vi "运维调试_质控单元.vi"() -> ()   [LabVIEW 2016, in "质控单元.lvlib"]
uses:
  <vilib>/Utility/miscctls.llb/LVPointTypeDef.ctl
  <vilib>/Utility/config.llb/Write Key (I32).vi
  <vilib>/Utility/config.llb/NI_LVConfig.lvlib
panel:
  in  "适用类型":enum16{"固定站", "微站"}(ring) caption="模块组合"
  in  "模块组合":enum16{"氨氮总磷", "总磷总氮", "氨氮、总磷、总氮"}(ring)=enum."氨氮、总磷、总氮"
  in  "解锁？":bool
  in  "锁定按钮":bool
  out "模块版本号":string
  out "CODCr加标后理论浓度":dbl format="%.2f"
  out "CODMn加标后理论浓度":dbl format="%.2f"
  out "总氮加标后理论浓度":dbl format="%.2f"
  out "总磷加标后理论浓度":dbl format="%.2f"
  out "氨氮加标后理论浓度":dbl format="%.2f"
  out "CODCr母液浓度":dbl caption="加标母液浓度" format="%.2f"
  out "CODCr加标水杯定容体积":dbl caption="加标水杯定容体积" format="%.2f"
  out "CODCr检出限":dbl caption="检出限" format="%.2f"
  out "CODCr量程":dbl caption="量程" format="%.2f"
  out "COD母液浓度":dbl caption="加标母液浓度" format="%.2f"
  out "COD加标水杯定容体积":dbl caption="加标水杯定容体积" format="%.2f"
  out "COD检出限":dbl caption="检出限" format="%.2f"
  out "COD量程":dbl caption="量程" format="%.2f"
  out "总氮母液浓度":dbl caption="加标母液浓度" format="%.3f"
  out "总氮加标水杯定容体积":dbl caption="加标水杯定容体积" format="%.2f"
  out "总氮检出限":dbl caption="检出限" format="%.3f"
  out "总氮量程":dbl caption="量程" format="%.2f"
  out "总磷母液浓度":dbl caption="加标母液浓度" format="%.3f"
  out "总磷加标水杯定容体积":dbl caption="加标水杯定容体积" format="%.2f"
  out "总磷检出限":dbl caption="检出限" format="%.3f"
  out "总磷量程":dbl caption="量程" format="%.2f"
  out "氨氮母液浓度":dbl caption="加标母液浓度" format="%.3f"
  out "氨氮加标水杯定容体积":dbl caption="加标水杯定容体积" format="%.2f"
  out "氨氮检出限":dbl caption="检出限" format="%.3f"
  out "氨氮量程":dbl caption="量程" format="%.2f"
  in  "流程读写":bool
  in  "隐藏按钮":bool
  in  "定时启动":bool
  out "串口/TCP":string
  out "CODCr状态簇":T1
  out "CODMn状态簇":T1
  out "总氮状态簇":T1
  out "总磷状态簇":T1
  out "氨氮状态簇":T1
  out "总氮柱塞泵故障报警":bool
  out "总氮液位异常报警":bool
  out "总氮液位状态":bool
  out "总氮流程中断报警":bool
  out "总氮质控流程中":bool caption="总磷质控流程中"
  out "总氮通讯":bool
  out "总氮加标回收率":dbl caption="加标回收率" format="%.2f"
  out "总氮加标体积":dbl caption="加标体积" format="%.3f"
  out "总氮加标后水样浓度":dbl caption="加标后水样浓度" format="%.3f"
  out "总氮加标前水样浓度":dbl caption="加标前水样浓度" format="%.3f"
  out "总氮状态":u16(ring) caption="状态" items=["待机", "润洗", "进样", "进样完成", "柱塞泵加标", "等待取液", "排液"]
  out "CODCr柱塞泵故障报警":bool
  out "CODCr质控流程中":bool
  out "CODCr通讯":bool
  out "CODCr传感器状态":bool
  out "CODCr传感器故障报警":bool
  out "CODCr流程中断报警":bool
  out "CODCr加标回收率":dbl caption="加标回收率" format="%.2f"
  out "CODCr加标体积":dbl caption="加标体积" format="%.3f"
  out "CODCr加标后水样浓度":dbl caption="加标后水样浓度" format="%.2f"
  out "CODCr加标前水样浓度":dbl caption="加标前水样浓度" format="%.2f"
  out "CODCr状态":u16(ring) caption="状态" items=["待机", "润洗", "进样", "进样完成", "柱塞泵加标", "等待取液", "排液"]
  out "CODMn柱塞泵故障报警":bool
  out "CODMn质控流程中":bool
  out "CODMn通讯":bool
  out "CODMn液位异常报警":bool
  out "CODMn液位状态":bool
  out "CODMn流程中断报警":bool
  out "COD加标回收率":dbl caption="加标回收率" format="%.2f"
  out "COD加标体积":dbl caption="加标体积" format="%.3f"
  out "COD加标后水样浓度":dbl caption="加标后水样浓度" format="%.2f"
  out "COD加标前水样浓度":dbl caption="加标前水样浓度" format="%.2f"
  out "CODMn状态":u16(ring) caption="状态" items=["待机", "润洗", "进样", "进样完成", "柱塞泵加标", "等待取液", "排液"]
  out "总磷柱塞泵故障报警":bool
  out "总磷通讯":bool
  out "总磷质控流程中":bool caption="总氮质控流程中"
  out "总磷液位异常报警":bool
  out "总磷液位状态":bool
  out "总磷流程中断报警":bool
  out "总磷加标回收率":dbl caption="加标回收率" format="%.2f"
  out "总磷加标体积":dbl caption="加标体积" format="%.3f"
  out "总磷加标后水样浓度":dbl caption="加标后水样浓度" format="%.3f"
  out "总磷加标前水样浓度":dbl caption="加标前水样浓度" format="%.3f"
  out "总磷状态":u16(ring) caption="状态" items=["待机", "润洗", "进样", "进样完成", "柱塞泵加标", "等待取液", "排液"]
  out "氨氮柱塞泵故障报警":bool
  out "氨氮质控流程中":bool
  out "氨氮通讯":bool
  out "氨氮液位异常报警":bool
  out "氨氮液位状态":bool
  out "氨氮流程中断报警":bool
  out "氨氮加标回收率":dbl caption="加标回收率" format="%.2f"
  out "氨氮加标体积":dbl caption="加标体积" format="%.3f"
  out "氨氮加标后水样浓度":dbl caption="加标后水样浓度" format="%.3f"
  out "氨氮加标前水样浓度":dbl caption="加标前水样浓度" format="%.3f"
  out "氨氮状态":u16(ring) caption="状态" items=["待机", "润洗", "进样", "进样完成", "柱塞泵加标", "等待取液", "排液"]
  in  "总氮模块选择":bool caption="总氮模块"
  in  "释放串口":bool
  in  "打开串口":bool
  in  "柱塞泵调试":bool
  in  "手动调试":bool
  in  "报警清除":bool
  in  "参数设置":bool
  in  "停止测量":bool
  in  "加标回收":bool
  in  "平行样测试":bool
  in  "CODCr加标回收":enum32{"H", "L", "AUTO"}(ring)
  in  "CODCr选择":bool caption="CODCr模块"
  out "质控流程中":bool
  in  "CODMn加标回收":enum32{"H", "L", "AUTO"}(ring)
  in  "总磷加标回收":enum32{"H", "L", "AUTO"}(ring)=enum."AUTO"
  in  "总氮加标回收":enum32{"H", "L", "AUTO"}(ring)=enum."AUTO"
  in  "氨氮加标回收":enum32{"H", "L", "AUTO"}(ring)=enum."AUTO"
  in  "CODMn选择":bool caption="CODMn模块"
  in  "总磷模块选择":bool caption="总磷模块"
  in  "氨氮模块":bool
  in  "背隙补偿步数 3":i32 min=0 max=2000
  in  "背隙补偿步数 2":i32 min=0 max=2000
  in  "背隙补偿步数":i32 min=0 max=2000
  in  "返回":bool
  out "COD平行样测完标志":bool
  out "氨氮总磷平行样测完标志":bool
  # "氨氮"
  # "总磷"
  # "总氮"
  # "CODMn"
  # "CODCr"
  # "参数配置区"
  # "总磷质控参数"
  # "2000步等于1mL\n100步等于0.05mL\n20步等于0.01mL\n2步等于0.001mL\n（初始默认100步）"
  # "柱塞泵调试区"
  # "加标后理论浓度"
  # "mg/L"
  # "mg/L"
  # "mg/L"
  # "mg/L"
  # "mg/L"
  # "CODCr质控参数"
  # "mg/L"
  # "mL"
  # "mg/L"
  # "mg/L"
  # "CODMn质控参数"
  # "mg/L"
  # "mL"
  # "mg/L"
  # "mg/L"
  # "总氮质控参数"
  # "mg/L"
  # "mg/L"
  # "mL"
  # "mg/L"
  # "mg/L"
  # "mL"
  # "mg/L"
  # "mg/L"
  # "氨氮质控参数"
  # "mg/L"
  # "mL"
  # "mg/L"
  # "mg/L"
  # "%"
  # "mL"
  # "mg/L"
  # "mg/L"
  # "%"
  # "mL"
  # "mg/L"
  # "mg/L"
  # "%"
  # "mL"
  # "mg/L"
  # "mg/L"
  # "%"
  # "mL"
  # "mg/L"
  # "mg/L"
  # "%"
  # "mL"
  # "mg/L"
  # "mg/L"
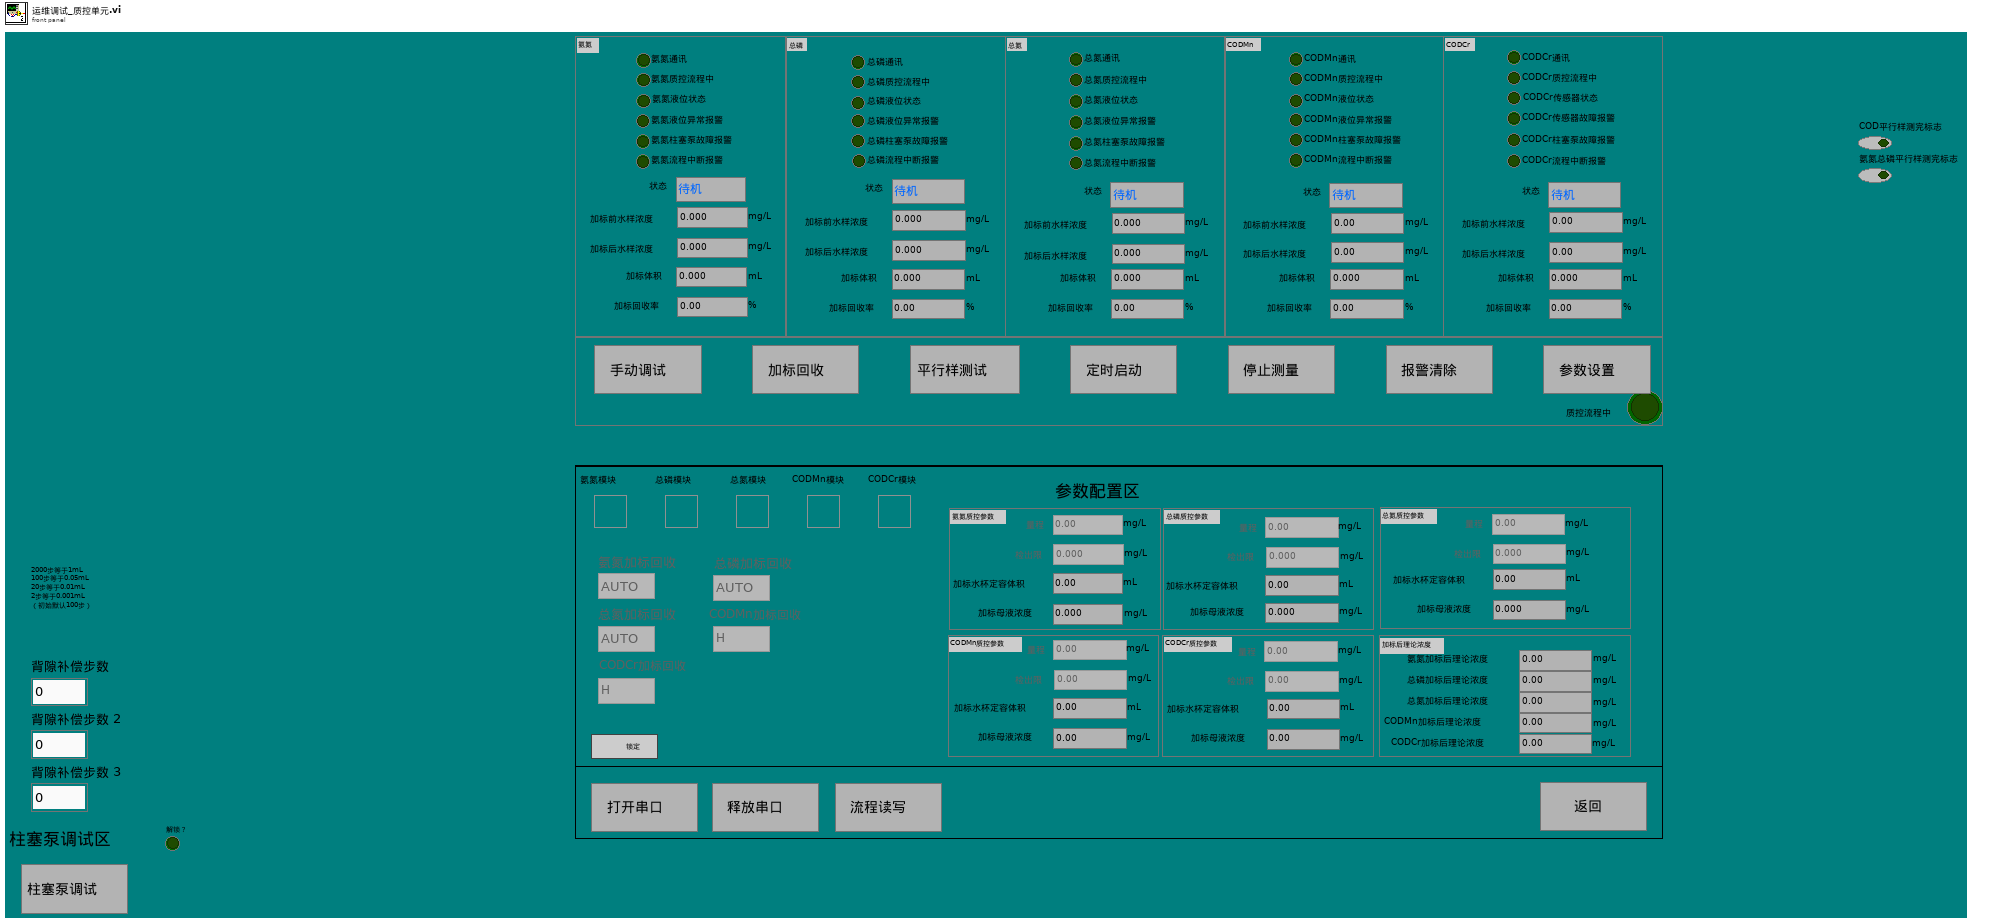
[diagram p1: front panel]
types:
  T1 = cluster{"步骤剩余时间":u16, "当前具体步骤":enum16{"加标", "进样", "排液", "搅拌", "定量"}, " 当前流程":enum16{"", "水样流程", "加标流程", "排液流程"}, "当前小步骤数":i8}
  T2 = typedef "LVPointTypeDef.ctl" = cluster{"Horizontal":i16, "Vertical":i16}
  T3 = cluster{"Major":u16, "Minor":u16, "Fix":u16, "Build":u16}
  T4 = cluster{"量程":dbl, "检出限":dbl, "加标前水样浓度":dbl, "加标后水样浓度":dbl, "加标水杯定容体积":dbl, "加标母液浓度":dbl, "加标体积":dbl, "加标回收率":dbl}
  T5 = cluster{"是否启用仪器":bool, "CODMn":cluster{"启动测量模式":cluster{"测量模式":enum16{"水样测量", "标样核查", "加标回收", "平行样", "校零", "校标"}}, "确定按钮":bool}, "启动模块":cluster{"氨氮":bool, "总磷":bool, "总氮":bool, "CODMn":bool, "CODCr":bool}, "常规启动":bool, "直接启动":bool}
  T6 = cluster{"参数启用":cluster{"CODMn":bool, "总磷":bool, "总氮":bool, "氨氮":bool, "CODcr":bool}, "采配水是否启动":bool}
  T7 = cluster{"命令":string, cluster{"starting address":u16, "holding register value":u16}}
  T8 = typedef "NI_LVConfig.lvlib/Config Data RefNum.ctl" = refnum<k1>
  T9 = cluster{"氨氮":bool, "总磷":bool, "总氮":bool, "CODMn":bool, "CODCr":bool}
  T10 = enum32{"Bad", "Idle", "Run top level", "Running"}
  T11 = cluster{"CODMn":bool, "总磷":bool, "总氮":bool, "氨氮":bool, "CODCr":bool}
  T12 = cluster{"周期设置类型":enum16{"定点启动", "间隔启动"}, "定时功能启用":bool, "定时间隔":dbl, "间隔启动次数 ":dbl, "已经启动次数 ":dbl, "24H周期设置":bool[], "模块选择":cluster{"氨氮":bool, "总磷":bool, "总氮":bool, "CODMn":bool, "CODCr":bool}, "采配水启用":bool}
  T13 = cluster{"周期设置类型":enum16{"定点启动", "间隔启动"}, "定时功能启用":bool, "定时间隔":dbl, "间隔启动次数":dbl, "已经启动次数":dbl, "24H周期设置":bool[], "模块选择":cluster{"氨氮":bool, "总磷":bool, "总氮":bool, "CODMn":bool, "CODCr":bool}, "采配水启用":bool}
  T14 = cluster{"氨氮":u8, "总磷":u8, "总氮":u8, "CODMn":u8, "CODCr":u8}
  T15 = enum8{"Enabled", "Disabled", "Disabled and Grayed Out"}
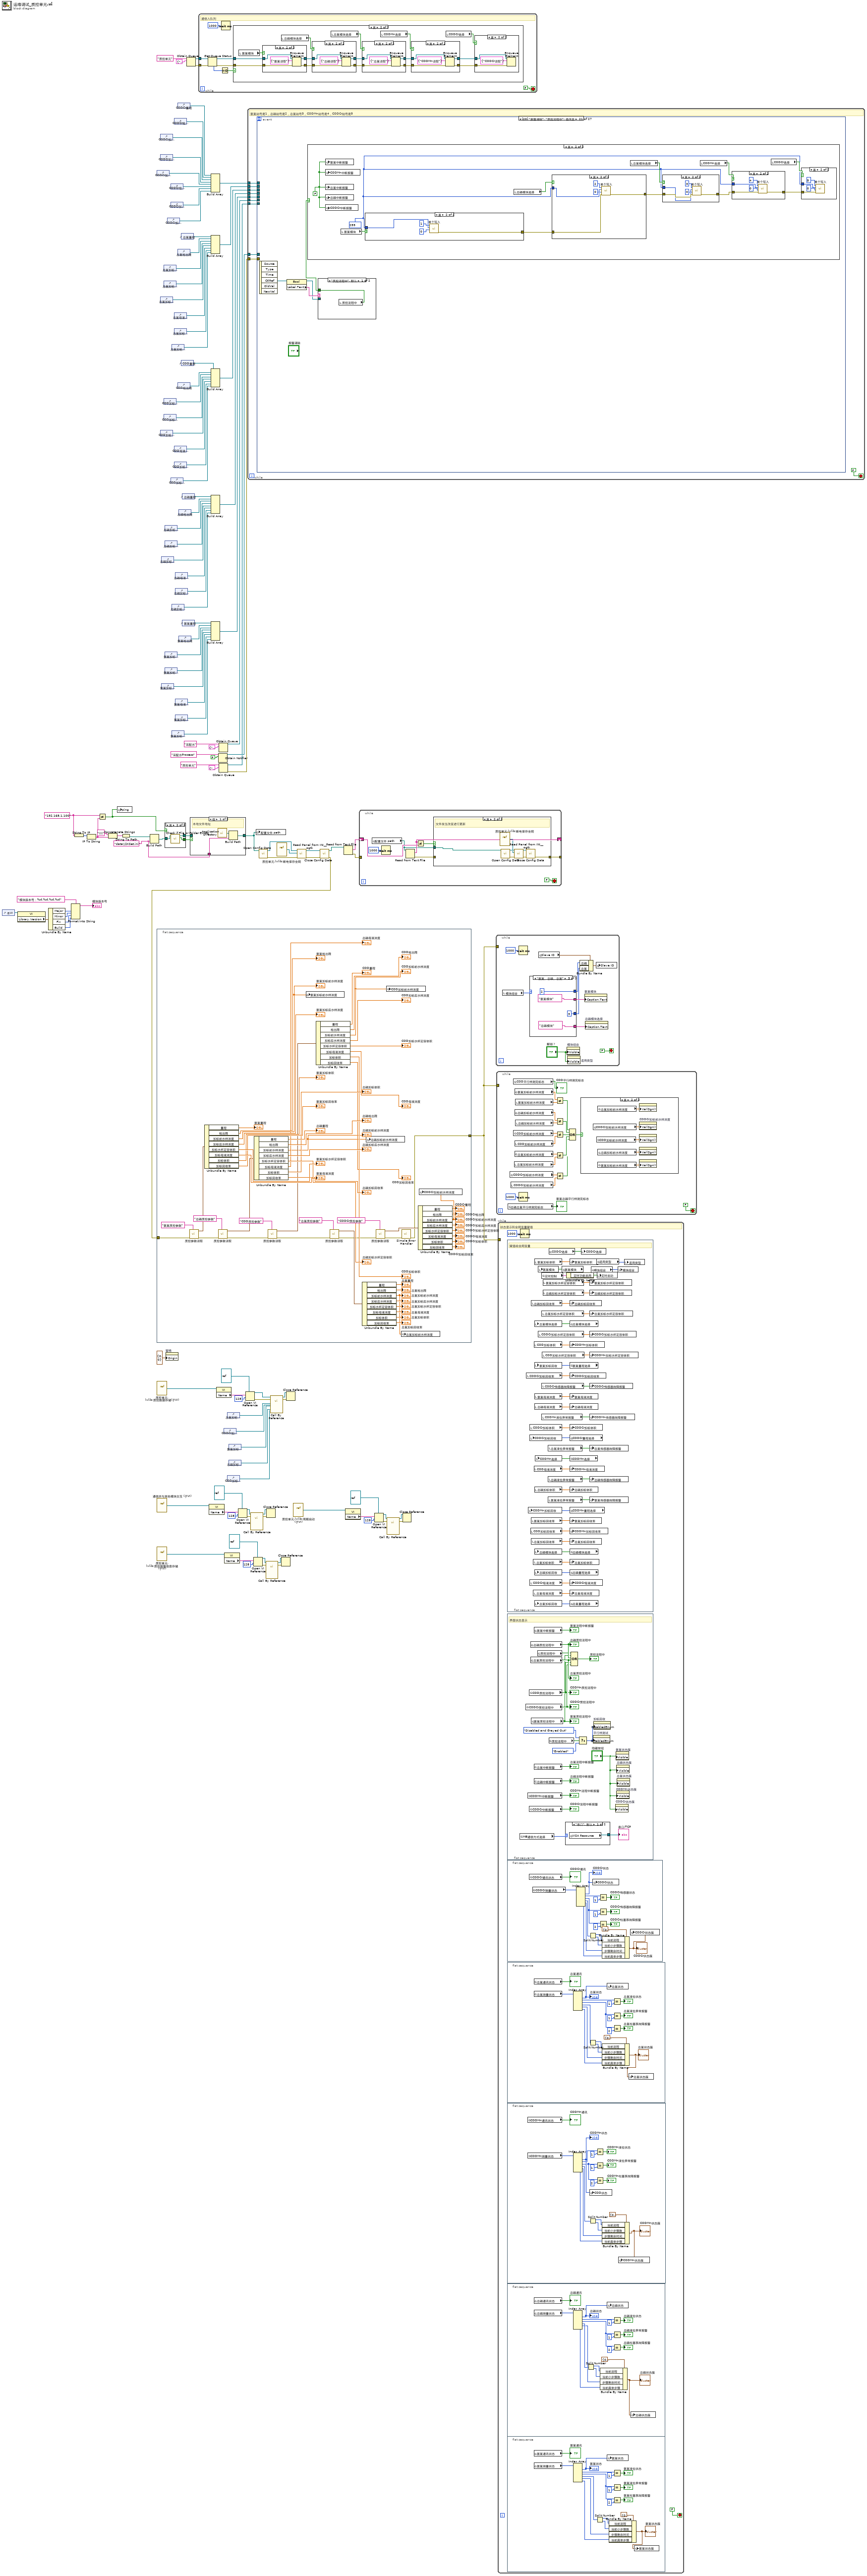
[diagram p0: block diagram]
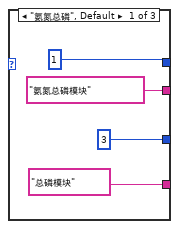
[diagram p2: hidden frame]
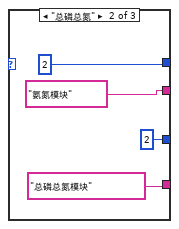
[diagram p3: hidden frame]
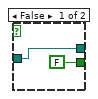
[diagram p4: hidden frame]
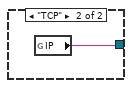
[diagram p13: hidden frame]
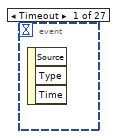
[diagram p15: hidden frame]
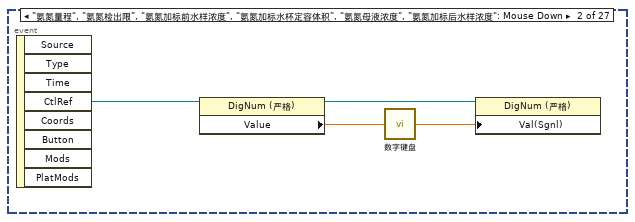
[diagram p16: hidden frame]
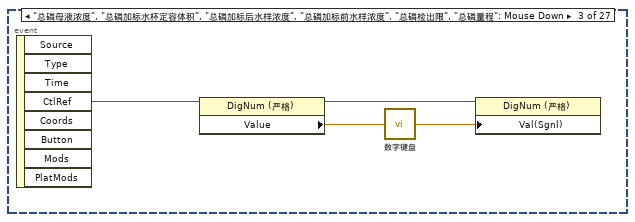
[diagram p17: hidden frame]
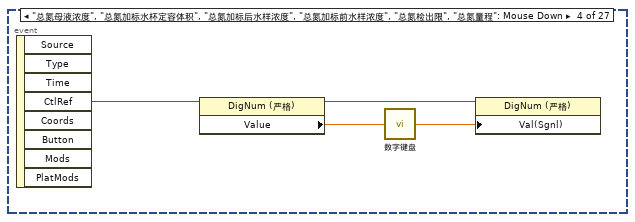
[diagram p18: hidden frame]
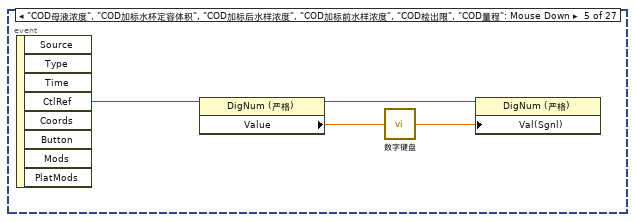
[diagram p19: hidden frame]
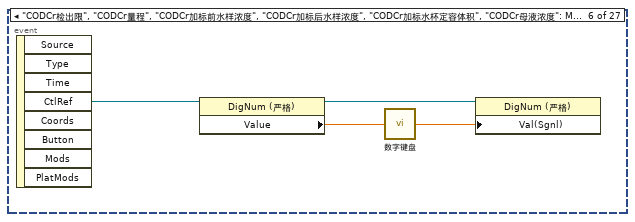
[diagram p20: hidden frame]
diagram:
  w30 = "data\\ZKSet.ini" ("名称或相对路径")
  w22 = "192.168.1.100" ("名称")
  n1 = control-ref of="本VI"() -> (w12:refnum<vi>)
  n2 = property class="VI"(reference=w12) -> ("Library.Version"=w11:T3)  [unwired: 1 in, 2 out]
  n3 = Unbundle By Name(w11) -> ("Major"=w9:u16, "Minor"=w8:u16, "Fix"=w7:u16, "Build"=w6:u16)
  n4 = Format Into String(format string="模块版本号：%d.%d.%d.%d" ("格式字符串"), w9, w8, w7, w6) -> (resulting string=→"模块版本号":string)  [unwired: 2 in, 1 out]
  n5 = String To IP(1:w22) -> (0:w29:u32)
  n6 = IP To String(2:w29) -> (0:w26:string)  [unwired: 1 in]
  n7 = Not Equal?(x=w22, y=w26) -> (x != y?=w21:bool)
  n8 = Concatenate Strings("\\\\" ("字符串"), w26) -> (w27:string)
  n9 = global write "质控内部交互全局.vi" "ping"(w21) -> ()
  n10 = String To Path(string=w27) -> (path=w3:path)
  n11 = Build Path(base path=w3, name or relative path=w30) -> (appended path=w25:path)
  n12 = control-ref of="CODCr加标水杯定容体积"() -> (w80:refnum<vi>)
  n13 = flat-sequence {
    tunnel: [w129] -> w1
    tunnel: w2 -> [w128]
    frame #0 {
      n14 = call "质控参数读取.vi"("section"="氨氮质控参数", "error in (no error)"=w128) -> ("error out"=w166:errorcluster, "参数"=w183:T4)  [unwired: 8 in]
      n15 = Unbundle By Name(w183) -> ("量程"=→"氨氮量程":dbl, "检出限"=→"氨氮检出限":dbl, "加标前水样浓度"=w134:dbl, "加标后水样浓度"=→"氨氮加标后水样浓度":dbl, "加标水杯定容体积"=→"氨氮加标水杯定容体积":dbl, "加标母液浓度"=→"氨氮母液浓度":dbl, "加标体积"=→"氨氮加标体积":dbl, "加标回收率"=→"氨氮加标回收率":dbl)
      "氨氮加标前水样浓度" <- w134
      n16 = call "质控参数读取.vi"("section"="总磷质控参数", "error in (no error)"=w166) -> ("error out"=w163:errorcluster, "参数"=w174:T4)  [unwired: 8 in]
      n17 = Unbundle By Name(w174) -> ("量程"=→"总磷量程":dbl, "检出限"=→"总磷检出限":dbl, "加标前水样浓度"=w133:dbl, "加标后水样浓度"=→"总磷加标后水样浓度":dbl, "加标水杯定容体积"=→"总磷加标水杯定容体积":dbl, "加标母液浓度"=→"总磷母液浓度":dbl, "加标体积"=→"总磷加标体积":dbl, "加标回收率"=→"总磷加标回收率":dbl)
      "总磷加标前水样浓度" <- w133
      n18 = call "质控参数读取.vi"("section"="COD质控参数", "error in (no error)"=w163) -> ("error out"=w154:errorcluster, "参数"=w165:T4)  [unwired: 8 in]
      n19 = global write "水样浓度全局.vi" "氨氮加标前水样浓度"(w134) -> ()
      n20 = Unbundle By Name(w165) -> ("量程"=→"COD量程":dbl, "检出限"=→"COD检出限":dbl, "加标前水样浓度"=w132:dbl, "加标后水样浓度"=→"COD加标后水样浓度":dbl, "加标水杯定容体积"=→"COD加标水杯定容体积":dbl, "加标母液浓度"=→"COD母液浓度":dbl, "加标体积"=→"COD加标体积":dbl, "加标回收率"=→"COD加标回收率":dbl)
      "COD加标前水样浓度" <- w132
      n21 = call "质控参数读取.vi"("section"="总氮质控参数", "error in (no error)"=w154) -> ("error out"=w143:errorcluster, "参数"=w153:T4)  [unwired: 8 in]
      n22 = Unbundle By Name(w153) -> ("量程"=→"总氮量程":dbl, "检出限"=→"总氮检出限":dbl, "加标前水样浓度"=w131:dbl, "加标后水样浓度"=→"总氮加标后水样浓度":dbl, "加标水杯定容体积"=→"总氮加标水杯定容体积":dbl, "加标母液浓度"=→"总氮母液浓度":dbl, "加标体积"=→"总氮加标体积":dbl, "加标回收率"=→"总氮加标回收率":dbl)
      "总氮加标前水样浓度" <- w131
      n23 = global write "水样浓度全局.vi" "总磷加标前水样浓度"(w133) -> ()
      n24 = call "质控参数读取.vi"("section"="CODCr质控参数", "error in (no error)"=w143) -> ("error out"=w135:errorcluster, "参数"=w144:T4)  [unwired: 8 in]
      n25 = global write "水样浓度全局.vi" "COD加标前水样浓度"(w132) -> ()
      n26 = global write "水样浓度全局.vi" "总氮加标前水样浓度"(w131) -> ()
      n27 = call <vilib>:"Simple Error Handler.vi"("error in (no error)"=w135) -> ("error out"=w129:errorcluster)  [unwired: 4 in, 4 out]
      n28 = Unbundle By Name(w144) -> ("量程"=→"CODCr量程":dbl, "检出限"=→"CODCr检出限":dbl, "加标前水样浓度"=w130:dbl, "加标后水样浓度"=→"CODCr加标后水样浓度":dbl, "加标水杯定容体积"=→"CODCr加标水杯定容体积":dbl, "加标母液浓度"=→"CODCr母液浓度":dbl, "加标体积"=→"CODCr加标体积":dbl, "加标回收率"=→"CODCr加标回收率":dbl)
      "CODCr加标前水样浓度" <- w130
      n29 = global write "水样浓度全局.vi" "CODCr加标前水样浓度"(w130) -> ()
    }
  }
  n30 = vi-ref "质控单元.lvlib:质控数据存储(子VI).vi"() -> (w55:refnum<vi>)
  n31 = vi-ref "通信并与其他模块交互 (子VI).vi"() -> (w68:refnum<vi>)
  n32 = vi-ref "质控单元.lvlib:质控报警信息存储 (子VI).vi"() -> (w63:refnum<vi>)
  n33 = control-ref of="CODCr加标前水样浓度"() -> (w82:refnum<vi>)
  n34 = control-ref of="CODCr加标后水样浓度"() -> (w81:refnum<vi>)
  n35 = control-ref of="总氮加标水杯定容体积"() -> (w89:refnum<vi>)
  n36 = control-ref of="COD加标水杯定容体积"() -> (w104:refnum<vi>)
  n37 = control-ref of="总磷加标水杯定容体积"() -> (w113:refnum<vi>)
  n38 = control-ref of="氨氮加标水杯定容体积"() -> (w123:refnum<vi>)
  n39 = control-ref of="总氮加标前水样浓度"() -> (w91:refnum<vi>)
  n40 = control-ref of="总氮加标后水样浓度"() -> (w90:refnum<vi>)
  n41 = control-ref of="COD加标前水样浓度"() -> (w106:refnum<vi>)
  n42 = control-ref of="COD加标后水样浓度"() -> (w105:refnum<vi>)
  n43 = control-ref of="总磷加标前水样浓度"() -> (w115:refnum<vi>)
  n44 = control-ref of="总磷加标后水样浓度"() -> (w114:refnum<vi>)
  n45 = control-ref of="氨氮加标前水样浓度"() -> (w124:refnum<vi>)
  n46 = control-ref of="氨氮加标后水样浓度"() -> (w120:refnum<vi>)
  n47 = case shown="真" w21 {
    tunnel: w25 -> [w185 w189]
    tunnel: [w185 w188] -> w24
    tunnel: [FALSE w187] -> w23
    frame False {
    }
    frame True {
      n48 = call <vilib>:"Check if File or Folder Exists.vi"("path"=w189) -> ("file or folder exists?"=w187:bool, "dup path"=w188:path)  [unwired: 8 in, 1 out]
    }
  }
  n49 = property on="窗格" class="Pane"("Origin"=T2 {"Horizontal"=0, "Vertical"=0} ("原点")) -> ()  [unwired: 2 in, 2 out]
  n50 = control-ref of="CODCr加标回收率"() -> (w77:refnum<vi>)
  n51 = control-ref of="CODCr母液浓度"() -> (w79:refnum<vi>)
  n52 = control-ref of="CODCr加标体积"() -> (w78:refnum<vi>)
  n53 = control-ref of="COD加标回收率"() -> (w101:refnum<vi>)
  n54 = control-ref of="总氮加标回收率"() -> (w86:refnum<vi>)
  n55 = control-ref of="总磷加标回收率"() -> (w111:refnum<vi>)
  n56 = control-ref of="氨氮加标回收率"() -> (w118:refnum<vi>)
  n57 = control-ref of="CODCr检出限"() -> (w83:refnum<vi>)
  n58 = control-ref of="总氮母液浓度"() -> (w88:refnum<vi>)
  n59 = control-ref of="总氮加标体积"() -> (w87:refnum<vi>)
  n60 = control-ref of="COD母液浓度"() -> (w103:refnum<vi>)
  n61 = control-ref of="COD加标体积"() -> (w102:refnum<vi>)
  n62 = control-ref of="总磷母液浓度"() -> (w112:refnum<vi>)
  n63 = control-ref of="总磷加标体积"() -> (w110:refnum<vi>)
  n64 = control-ref of="氨氮母液浓度"() -> (w122:refnum<vi>)
  n65 = control-ref of="氨氮加标体积"() -> (w119:refnum<vi>)
  n66 = control-ref of="CODCr量程"() -> (w84:refnum<vi>)
  n67 = control-ref of="总氮检出限"() -> (w92:refnum<vi>)
  n68 = control-ref of="COD检出限"() -> (w107:refnum<vi>)
  n69 = control-ref of="总磷检出限"() -> (w116:refnum<vi>)
  n70 = control-ref of="氨氮检出限"() -> (w125:refnum<vi>)
  n71 = control-ref of="总氮量程"() -> (w93:refnum<vi>)
  n72 = control-ref of="COD量程"() -> (w108:refnum<vi>)
  n73 = control-ref of="总磷量程"() -> (w117:refnum<vi>)
  n74 = control-ref of="氨氮量程"() -> (w126:refnum<vi>)
  n75 = Obtain Queue(name (unnamed)="质控单元" ("名称（未命名）"), element data type=cluster{"命令":string} {"命令"="启用模块"} ("元素")) -> (queue out=w40:refnum<queue>, error out=w39:errorcluster)  [unwired: 3 in, 1 out]
  n76 = case shown="假" w23 {
    tunnel: w24 -> [_ w193]
    tunnel: [w191 w193] -> w14
    tunnel: w30 -> [w190 _]
    frame False {
      # "本地文件地址"
      n77 = call <vilib>:"Application Directory.vi"() -> ("Application Directory"=w192:path)
      n78 = Build Path(base path=w192, name or relative path=w190) -> (appended path=w191:path)
    }
    frame True {
      # "网络共享地址"
    }
  }
  n79 = while {
    tunnel: w40 -> [w199]
    tunnel: w39 -> [w198]
    stop <- FALSE stop-if-true
    # "通信入队列"
    n80 = Get Queue Status(queue=w199, error in (no error)=w198) -> (queue out=w196:refnum<queue>, error out=w195:errorcluster, # elements in queue=w197:i32)  [unwired: 1 in, 5 out]
    n81 = Equal To 0?(x=w197) -> (x = 0?=w194:bool)
    n82 = Wait (ms)(milliseconds to wait=u32 1000 ("等待时间（毫秒）")) -> ()  [unwired: 1 out]
    n83 = case shown="真" w194 {
      tunnel: w196 -> [_ w216]
      tunnel: w195 -> [_ w215]
      frame False {
      }
      frame True {
        n84 = local read "氨氮模块"() -> (w214:bool)
        n85 = case shown="真" w214 {
          tunnel: w216 -> [w242 w246]
          tunnel: w215 -> [w241 w245]
          tunnel: [w242 w244] -> w212
          tunnel: [w241 w243] -> w211
          frame False {
          }
          frame True {
            n86 = Enqueue Element(queue=w246, element=cluster{"命令":string} {"命令"="氨氮读取"} ("元素"), error in (no error)=w245) -> (queue out=w244:refnum<queue>, error out=w243:errorcluster)  [unwired: 1 in, 1 out]
          }
        }
        n87 = local read "总磷模块选择"() -> (w213:bool)
        n88 = case shown="真" w213 {
          tunnel: w212 -> [w235 w239]
          tunnel: w211 -> [w234 w238]
          tunnel: [w235 w237] -> w209
          tunnel: [w234 w236] -> w208
          frame False {
          }
          frame True {
            n89 = Enqueue Element(queue=w239, element=cluster{"命令":string} {"命令"="总磷读取"} ("元素"), error in (no error)=w238) -> (queue out=w237:refnum<queue>, error out=w236:errorcluster)  [unwired: 1 in, 1 out]
          }
        }
        n90 = local read "总氮模块选择"() -> (w210:bool)
        n91 = case shown="真" w210 {
          tunnel: w209 -> [w228 w232]
          tunnel: w208 -> [w227 w231]
          tunnel: [w228 w230] -> w206
          tunnel: [w227 w229] -> w205
          frame False {
          }
          frame True {
            n92 = Enqueue Element(queue=w232, element=cluster{"命令":string} {"命令"="总氮读取"} ("元素"), error in (no error)=w231) -> (queue out=w230:refnum<queue>, error out=w229:errorcluster)  [unwired: 1 in, 1 out]
          }
        }
        n93 = local read "CODMn选择"() -> (w207:bool)
        n94 = case shown="真" w207 {
          tunnel: w206 -> [w221 w225]
          tunnel: w205 -> [w220 w224]
          tunnel: [w221 w223] -> w203
          tunnel: [w220 w222] -> w202
          frame False {
          }
          frame True {
            n95 = Enqueue Element(queue=w225, element=cluster{"命令":string} {"命令"="CODMn读取"} ("元素"), error in (no error)=w224) -> (queue out=w223:refnum<queue>, error out=w222:errorcluster)  [unwired: 1 in, 1 out]
          }
        }
        n96 = local read "CODCr选择"() -> (w204:bool)
        n97 = case shown="真" w204 {
          tunnel: w203 -> [_ w218]
          tunnel: w202 -> [_ w217]
          frame False {
          }
          frame True {
            n98 = Enqueue Element(queue=w218, element=cluster{"命令":string} {"命令"="CODCr读取"} ("元素"), error in (no error)=w217) -> ()  [unwired: 1 in, 3 out]
          }
        }
      }
    }
  }
  n99 = property class="VI"(reference=w68) -> ("Name"=w69:string)  [unwired: 1 in, 2 out]
  n100 = Build Array(w84, w83, w82, w81, w80, w79, w78, w77) -> (w76:refnum<vi>[])
  n101 = Build Array(w93, w92, w91, w90, w89, w88, w87, w86) -> (w85:refnum<vi>[])
  n102 = Build Array(w108, w107, w106, w105, w104, w103, w102, w101) -> (w100:refnum<vi>[])
  n103 = Build Array(w117, w116, w115, w114, w113, w112, w110, w111) -> (w109:refnum<vi>[])
  n104 = Build Array(w126, w125, w124, w120, w123, w122, w119, w118) -> (w121:refnum<vi>[])
  n105 = property class="VI"(reference=w55) -> ("Name"=w54:string)  [unwired: 1 in, 2 out]
  n106 = Obtain Notifier(name (unnamed)="采配水Process" ("名称（未命名）"), notification data type=FALSE) -> (notifier out=w97:refnum<notifier>)  [unwired: 2 in, 2 out]
  n107 = Obtain Queue(name (unnamed)="采配水" ("名称（未命名）"), element data type=cluster{"命令":string, "数据":variant} {"命令"="", "数据"=variant}) -> (queue out=w94:refnum<queue>)  [unwired: 3 in, 2 out]
  n108 = Obtain Queue(name (unnamed)="质控单元" ("名称（未命名）"), element data type=cluster{"命令":string} {"命令"="启用模块"} ("元素")) -> (queue out=w65:refnum<queue>, error out=w64:errorcluster)  [unwired: 3 in, 1 out]
  n109 = control-ref of="CODCr加标后水样浓度"() -> (w43:refnum<vi>)
  n110 = property class="VI"(reference=w63) -> ("Name"=w62:string)  [unwired: 1 in, 2 out]
  n111 = control-ref of="总氮加标后水样浓度"() -> (w47:refnum<vi>)
  n112 = control-ref of="COD加标后水样浓度"() -> (w44:refnum<vi>)
  n113 = control-ref of="氨氮加标后水样浓度"() -> (w46:refnum<vi>)
  n114 = control-ref of="总磷加标后水样浓度"() -> (w45:refnum<vi>)
  n115 = Open VI Reference(type specifier VI Refnum (for type only)=refnum<vi> refnum, vi path=w69, options=128 ("选项")) -> (vi reference=w71:refnum<vi>, error out=w73:errorcluster)  [unwired: 3 in]
  n116 = Open VI Reference(type specifier VI Refnum (for type only)=refnum<vi> refnum, vi path=w54, options=128 ("选项")) -> (vi reference=w52:refnum<vi>, error out=w50:errorcluster)  [unwired: 3 in]
  n117 = while {
    tunnel: w121 -> [w256]
    tunnel: w109 -> [w255]
    tunnel: w100 -> [w250]
    tunnel: w97 -> [w254]
    tunnel: w94 -> [w253]
    tunnel: w85 -> [w252]
    tunnel: w76 -> [w251]
    tunnel: w65 -> [w249]
    tunnel: w64 -> [w248]
    stop <- FALSE stop-if-true
    # "氨氮站号是1，总磷站号是2，总氮站号3，CODMn站号是4，CODCr站号是5"
    n118 = event shown="[20] \"报警清除\", \"质控流程中\": 值改变" {
      selector: _ -> [_ _ _ _ _ _ _ _ _ _ _ _ _ _ _ _ _ _ _ _ _ _ _ _ _ _ _]
      dyn-events: _ -> [_ _ _ _ _ _ _ _ _ _ _ _ _ _ _ _ _ _ _ _ _ _ _ _ _ _ _]
      timeout: _ -> [_ _ _ _ _ _ _ _ _ _ _ _ _ _ _ _ _ _ _ _ _ _ _ _ _ _ _]
      tunnel: w256 -> [_ _ _ _ _ _ _ _ _ w312 _ _ _ _ _ _ _ _ _ _ _ _ _ _ _ _ _]
      tunnel: w255 -> [_ _ _ _ _ _ _ _ _ _ w327 _ _ _ _ _ _ _ _ _ _ _ _ _ _ _ _]
      tunnel: w250 -> [_ _ _ _ _ _ _ _ _ _ _ _ w367 _ _ _ _ _ _ _ _ _ _ _ _ _ _]
      tunnel: w254 -> [_ _ _ _ _ _ _ _ _ _ _ _ _ _ _ _ _ _ _ w446 _ w527 w543 _ _ _ _]
      tunnel: w253 -> [_ _ _ _ _ _ _ _ _ _ _ _ _ _ _ _ _ _ _ _ _ _ w544 _ _ _ _]
      tunnel: w252 -> [_ _ _ _ _ _ _ _ _ _ _ w346 _ _ _ _ _ _ _ _ _ _ _ _ _ _ _]
      tunnel: w251 -> [_ _ _ _ _ _ _ _ _ _ _ _ _ w386 _ _ _ _ _ _ _ _ _ _ _ _ _]
      tunnel: w249 -> [_ _ _ _ _ _ _ _ _ _ _ _ _ _ _ _ _ w410 w430 _ _ _ _ _ _ _ _]
      tunnel: w248 -> [_ _ _ _ _ _ _ _ _ _ _ _ _ _ _ _ _ w409 w429 _ _ _ _ _ _ _ _]
      event Timeout {
        n119 = event-data() -> ()  [unwired: 1 in, 3 out]
      }
      event "氨氮量程", "氨氮检出限", "氨氮加标前水样浓度", "氨氮加标水杯定容体积", "氨氮母液浓度", "氨氮加标后水样浓度": Mouse Down {
        n120 = event-data() -> ("CtlRef"=w261:refnum<vi>)  [unwired: 1 in, 7 out]
        n121 = property class="DigNum (严格)"(reference=w261) -> (reference out=w259:refnum<vi>, "Value"=w260:dbl)  [unwired: 1 in, 1 out]
        n122 = call "数字键盘.vi"("OldNumber"=w260) -> ("NewNumber"=w258:sgl)
        n123 = property class="DigNum (严格)"(reference=w259, "Val(Sgnl)"=w258) -> ()  [unwired: 1 in, 2 out]
      }
      event "总磷母液浓度", "总磷加标水杯定容体积", "总磷加标后水样浓度", "总磷加标前水样浓度", "总磷检出限", "总磷量程": Mouse Down {
        n124 = event-data() -> ("CtlRef"=w265:refnum<vi>)  [unwired: 1 in, 7 out]
        n125 = property class="DigNum (严格)"(reference=w265) -> (reference out=w263:refnum<vi>, "Value"=w264:dbl)  [unwired: 1 in, 1 out]
        n126 = call "数字键盘.vi"("OldNumber"=w264) -> ("NewNumber"=w262:sgl)
        n127 = property class="DigNum (严格)"(reference=w263, "Val(Sgnl)"=w262) -> ()  [unwired: 1 in, 2 out]
      }
      event "总氮母液浓度", "总氮加标水杯定容体积", "总氮加标后水样浓度", "总氮加标前水样浓度", "总氮检出限", "总氮量程": Mouse Down {
        n128 = event-data() -> ("CtlRef"=w269:refnum<vi>)  [unwired: 1 in, 7 out]
        n129 = property class="DigNum (严格)"(reference=w269) -> (reference out=w267:refnum<vi>, "Value"=w268:dbl)  [unwired: 1 in, 1 out]
        n130 = call "数字键盘.vi"("OldNumber"=w268) -> ("NewNumber"=w266:sgl)
        n131 = property class="DigNum (严格)"(reference=w267, "Val(Sgnl)"=w266) -> ()  [unwired: 1 in, 2 out]
      }
      event "COD母液浓度", "COD加标水杯定容体积", "COD加标后水样浓度", "COD加标前水样浓度", "COD检出限", "COD量程": Mouse Down {
        n132 = event-data() -> ("CtlRef"=w273:refnum<vi>)  [unwired: 1 in, 7 out]
        n133 = property class="DigNum (严格)"(reference=w273) -> (reference out=w271:refnum<vi>, "Value"=w272:dbl)  [unwired: 1 in, 1 out]
        n134 = call "数字键盘.vi"("OldNumber"=w272) -> ("NewNumber"=w270:sgl)
        n135 = property class="DigNum (严格)"(reference=w271, "Val(Sgnl)"=w270) -> ()  [unwired: 1 in, 2 out]
      }
      event "CODCr检出限", "CODCr量程", "CODCr加标前水样浓度", "CODCr加标后水样浓度", "CODCr加标水杯定容体积", "CODCr母液浓度": Mouse Down {
        n136 = event-data() -> ("CtlRef"=w274:refnum<vi>)  [unwired: 1 in, 7 out]
        n137 = property class="DigNum (严格)"(reference=w274) -> (reference out=w276:refnum<vi>, "Value"=w277:dbl)  [unwired: 1 in, 1 out]
        n138 = call "数字键盘.vi"("OldNumber"=w277) -> ("NewNumber"=w275:sgl)
        n139 = property class="DigNum (严格)"(reference=w276, "Val(Sgnl)"=w275) -> ()  [unwired: 1 in, 2 out]
      }
      event "背隙补偿步数", "背隙补偿步数 2", "背隙补偿步数 3": Mouse Down {
        n140 = event-data() -> ("CtlRef"=w281:refnum<vi>)  [unwired: 1 in, 7 out]
        n141 = property class="DigNum (严格)"(reference=w281) -> (reference out=w280:refnum<vi>, "Value"=w279:i32)  [unwired: 1 in, 1 out]
        n142 = call "数字键盘.vi"("OldNumber"=w279) -> ("NewNumber"=w278:sgl)
        n143 = property class="DigNum (严格)"(reference=w280, "Val(Sgnl)"=w278) -> ()  [unwired: 1 in, 2 out]
      }
      event "背隙补偿步数", "背隙补偿步数 2", "背隙补偿步数 3": Value Change {
        w290 = "质控背隙补偿" ("section")
        n144 = event-data() -> ()  [unwired: 1 in, 6 out]
        n145 = call <vilib>:"Application Directory.vi"() -> ("Application Directory"=w297:path)
        n146 = Build Path(base path=w297, name or relative path="data\\Set.ini" ("名称或相对路径")) -> (appended path=w295:path)
        n147 = call <vilib>:"Open Config Data.vi"("configuration file path"=w295) -> ("error out"=w293:errorcluster, "refnum"=w294:T8)  [unwired: 8 in, 1 out]
        n148 = call-poly <vilib>:"Write Key.vi"("section"=w290, "error in (no error)"=w293, "value"="背隙补偿步数", "key"="背隙值1", "refnum"=w294) -> ("error out"=w284:errorcluster, "refnum out"=w287:T8)  [unwired: 4 in, 1 out]
        n149 = call-poly <vilib>:"Write Key.vi"("section"=w290, "error in (no error)"=w284, "value"="背隙补偿步数 2", "key"="背隙值2", "refnum"=w287) -> ("error out"=w285:errorcluster, "refnum out"=w286:T8)  [unwired: 4 in, 1 out]
        n150 = call-poly <vilib>:"Write Key.vi"("section"=w290, "error in (no error)"=w285, "value"="背隙补偿步数 3", "key"="背隙值3", "refnum"=w286) -> ()  [unwired: 4 in, 3 out]
      }
      event "氨氮模块", "总磷模块选择", "CODMn选择", "CODCr选择", "总氮模块选择", "模块组合", "适用类型": Value Change {
        n151 = event-data() -> ()  [unwired: 1 in, 6 out]
        n152 = flat-sequence {
          frame #0 {
            n153 = global write "断电保存全局.vi" "总磷模块选择"("总磷模块选择") -> ()
            n154 = global write "断电保存全局.vi" "模块组合"("模块组合") -> ()
            n155 = global write "断电保存全局.vi" "适用类型"("适用类型") -> ()
            n156 = global write "断电保存全局.vi" "总氮模块选择"("总氮模块选择") -> ()
            n157 = global write "断电保存全局.vi" "CODCr选择"("CODCr选择") -> ()
            n158 = global write "断电保存全局.vi" "CODMn选择"("CODMn选择") -> ()
            n159 = global write "断电保存全局.vi" "氨氮模块"("氨氮模块") -> ()
          }
          frame #1 {
            n160 = call "配置文件保存.vi"() -> ()  [unwired: 12 in]
          }
        }
      }
      event "氨氮量程", "氨氮检出限", "氨氮加标前水样浓度", "氨氮母液浓度", "氨氮加标水杯定容体积", "氨氮加标后水样浓度": Value Change {
        n161 = event-data() -> ()  [unwired: 1 in, 6 out]
        n162 = for {
          tunnel: w312 -> [w324] mode=indexing
          tunnel: [w323] -> w321 mode=indexing
          n163 = property class="DigNum (严格)"(reference=w324) -> ("Value"=w323:dbl)  [unwired: 1 in, 2 out]
        }
        n164 = Index Array(array=w321) -> (element #1=w320:dbl, element #2=w319:dbl, element #3=w306:dbl, element #4=w318:dbl, element #5=w317:dbl, element #6=w315:dbl)  [unwired: 6 in]
        n165 = global write "水样浓度全局.vi" "氨氮加标前水样浓度"(w306) -> ()
        n166 = Bundle By Name(cluster=T4 {"量程"=0.0, "检出限"=0.0, "加标前水样浓度"=0.0, "加标后水样浓度"=0.0, "加标水杯定容体积"=0.0, "加标母液浓度"=0.0, "加标体积"=0.0, "加标回收率"=0.0} ("参数"), "量程"=w320, "检出限"=w319, "加标前水样浓度"=w306, "加标后水样浓度"=w318, "加标水杯定容体积"=w317, "加标母液浓度"=w315) -> (w314:T4)
        n167 = call "加标回收率计算.vi"("参数"=w314) -> ("加标后理论浓度"=→"氨氮加标后理论浓度":dbl, "参数 out"=w313:T4)  [unwired: 9 in]
        n168 = call "质控参数保存.vi"("section"="氨氮质控参数", "参数"=w313) -> ()  [unwired: 9 in, 1 out]
        n169 = Unbundle By Name(w313) -> ("加标体积"=w307:dbl, "加标回收率"=w308:dbl)
        n170 = Index Array(array=w312, index #1=6 ("索引")) -> (element #1=w311:refnum<vi>, element #2=w309:refnum<vi>)  [unwired: 1 in]
        n171 = property class="DigNum (严格)"(reference=w311, "Value"=w307) -> ()  [unwired: 1 in, 2 out]
        n172 = property class="DigNum (严格)"(reference=w309, "Value"=w308) -> ()  [unwired: 1 in, 2 out]
      }
      event "总磷母液浓度", "总磷加标水杯定容体积", "总磷加标后水样浓度", "总磷加标前水样浓度", "总磷检出限", "总磷量程": Value Change {
        n173 = event-data() -> ()  [unwired: 1 in, 6 out]
        n174 = for {
          tunnel: w327 -> [w344] mode=indexing
          tunnel: [w343] -> w341 mode=indexing
          n175 = property class="DigNum (严格)"(reference=w344) -> ("Value"=w343:dbl)  [unwired: 1 in, 2 out]
        }
        n176 = Index Array(array=w341) -> (element #1=w340:dbl, element #2=w339:dbl, element #3=w326:dbl, element #4=w338:dbl, element #5=w337:dbl, element #6=w335:dbl)  [unwired: 6 in]
        n177 = global write "水样浓度全局.vi" "总磷加标前水样浓度"(w326) -> ()
        n178 = Bundle By Name(cluster=T4 {"量程"=0.0, "检出限"=0.0, "加标前水样浓度"=0.0, "加标后水样浓度"=0.0, "加标水杯定容体积"=0.0, "加标母液浓度"=0.0, "加标体积"=0.0, "加标回收率"=0.0} ("参数"), "量程"=w340, "检出限"=w339, "加标前水样浓度"=w326, "加标后水样浓度"=w338, "加标水杯定容体积"=w337, "加标母液浓度"=w335) -> (w334:T4)
        n179 = call "加标回收率计算.vi"("参数"=w334) -> ("加标后理论浓度"=→"总磷加标后理论浓度":dbl, "参数 out"=w333:T4)  [unwired: 9 in]
        n180 = call "质控参数保存.vi"("section"="总磷质控参数", "参数"=w333) -> ()  [unwired: 9 in, 1 out]
        n181 = Unbundle By Name(w333) -> ("加标体积"=w330:dbl, "加标回收率"=w328:dbl)
        n182 = Index Array(array=w327, index #1=6 ("索引")) -> (element #1=w332:refnum<vi>, element #2=w329:refnum<vi>)  [unwired: 1 in]
        n183 = property class="DigNum (严格)"(reference=w332, "Value"=w330) -> ()  [unwired: 1 in, 2 out]
        n184 = property class="DigNum (严格)"(reference=w329, "Value"=w328) -> ()  [unwired: 1 in, 2 out]
      }
      event "总氮量程", "总氮检出限", "总氮加标前水样浓度", "总氮加标后水样浓度", "总氮加标水杯定容体积", "总氮母液浓度": Value Change {
        n185 = event-data() -> ()  [unwired: 1 in, 6 out]
        n186 = for {
          tunnel: w346 -> [w364] mode=indexing
          tunnel: [w363] -> w361 mode=indexing
          n187 = property class="DigNum (严格)"(reference=w364) -> ("Value"=w363:dbl)  [unwired: 1 in, 2 out]
        }
        n188 = Index Array(array=w361) -> (element #1=w360:dbl, element #2=w359:dbl, element #3=w347:dbl, element #4=w358:dbl, element #5=w357:dbl, element #6=w355:dbl)  [unwired: 6 in]
        n189 = global write "水样浓度全局.vi" "总氮加标前水样浓度"(w347) -> ()
        n190 = Bundle By Name(cluster=T4 {"量程"=0.0, "检出限"=0.0, "加标前水样浓度"=0.0, "加标后水样浓度"=0.0, "加标水杯定容体积"=0.0, "加标母液浓度"=0.0, "加标体积"=0.0, "加标回收率"=0.0} ("参数"), "量程"=w360, "检出限"=w359, "加标前水样浓度"=w347, "加标后水样浓度"=w358, "加标水杯定容体积"=w357, "加标母液浓度"=w355) -> (w354:T4)
        n191 = call "加标回收率计算.vi"("参数"=w354) -> ("加标后理论浓度"=→"总氮加标后理论浓度":dbl, "参数 out"=w353:T4)  [unwired: 9 in]
        n192 = call "质控参数保存.vi"("section"="总氮质控参数", "参数"=w353) -> ()  [unwired: 9 in, 1 out]
        n193 = Unbundle By Name(w353) -> ("加标体积"=w350:dbl, "加标回收率"=w348:dbl)
        n194 = Index Array(array=w346, index #1=6 ("索引")) -> (element #1=w352:refnum<vi>, element #2=w349:refnum<vi>)  [unwired: 1 in]
        n195 = property class="DigNum (严格)"(reference=w352, "Value"=w350) -> ()  [unwired: 1 in, 2 out]
        n196 = property class="DigNum (严格)"(reference=w349, "Value"=w348) -> ()  [unwired: 1 in, 2 out]
      }
      event "COD母液浓度", "COD加标水杯定容体积", "COD加标后水样浓度", "COD加标前水样浓度", "COD检出限", "COD量程": Value Change {
        n197 = event-data() -> ()  [unwired: 1 in, 6 out]
        n198 = for {
          tunnel: w367 -> [w384] mode=indexing
          tunnel: [w383] -> w381 mode=indexing
          n199 = property class="DigNum (严格)"(reference=w384) -> ("Value"=w383:dbl)  [unwired: 1 in, 2 out]
        }
        n200 = Index Array(array=w381) -> (element #1=w380:dbl, element #2=w379:dbl, element #3=w366:dbl, element #4=w378:dbl, element #5=w377:dbl, element #6=w375:dbl)  [unwired: 6 in]
        n201 = global write "水样浓度全局.vi" "COD加标前水样浓度"(w366) -> ()
        n202 = Bundle By Name(cluster=T4 {"量程"=0.0, "检出限"=0.0, "加标前水样浓度"=0.0, "加标后水样浓度"=0.0, "加标水杯定容体积"=0.0, "加标母液浓度"=0.0, "加标体积"=0.0, "加标回收率"=0.0} ("参数"), "量程"=w380, "检出限"=w379, "加标前水样浓度"=w366, "加标后水样浓度"=w378, "加标水杯定容体积"=w377, "加标母液浓度"=w375) -> (w374:T4)
        n203 = call "加标回收率计算.vi"("参数"=w374) -> ("加标后理论浓度"=→"CODMn加标后理论浓度":dbl, "参数 out"=w373:T4)  [unwired: 9 in]
        n204 = call "质控参数保存.vi"("section"="COD质控参数", "参数"=w373) -> ()  [unwired: 9 in, 1 out]
        n205 = Unbundle By Name(w373) -> ("加标体积"=w370:dbl, "加标回收率"=w368:dbl)
        n206 = Index Array(array=w367, index #1=6 ("索引")) -> (element #1=w372:refnum<vi>, element #2=w369:refnum<vi>)  [unwired: 1 in]
        n207 = property class="DigNum (严格)"(reference=w372, "Value"=w370) -> ()  [unwired: 1 in, 2 out]
        n208 = property class="DigNum (严格)"(reference=w369, "Value"=w368) -> ()  [unwired: 1 in, 2 out]
      }
      event "CODCr母液浓度", "CODCr加标水杯定容体积", "CODCr加标前水样浓度", "CODCr检出限", "CODCr量程", "CODCr加标后水样浓度": Value Change {
        n209 = event-data() -> ()  [unwired: 1 in, 6 out]
        n210 = for {
          tunnel: w386 -> [w404] mode=indexing
          tunnel: [w403] -> w401 mode=indexing
          n211 = property class="DigNum (严格)"(reference=w404) -> ("Value"=w403:dbl)  [unwired: 1 in, 2 out]
        }
        n212 = Index Array(array=w401) -> (element #1=w400:dbl, element #2=w399:dbl, element #3=w387:dbl, element #4=w398:dbl, element #5=w397:dbl, element #6=w395:dbl)  [unwired: 6 in]
        n213 = global write "水样浓度全局.vi" "CODCr加标前水样浓度"(w387) -> ()
        n214 = Bundle By Name(cluster=T4 {"量程"=0.0, "检出限"=0.0, "加标前水样浓度"=0.0, "加标后水样浓度"=0.0, "加标水杯定容体积"=0.0, "加标母液浓度"=0.0, "加标体积"=0.0, "加标回收率"=0.0} ("参数"), "量程"=w400, "检出限"=w399, "加标前水样浓度"=w387, "加标后水样浓度"=w398, "加标水杯定容体积"=w397, "加标母液浓度"=w395) -> (w394:T4)
        n215 = call "加标回收率计算.vi"("参数"=w394) -> ("加标后理论浓度"=→"CODCr加标后理论浓度":dbl, "参数 out"=w393:T4)  [unwired: 9 in]
        n216 = call "质控参数保存.vi"("section"="CODCr质控参数", "参数"=w393) -> ()  [unwired: 9 in, 1 out]
        n217 = Unbundle By Name(w393) -> ("加标体积"=w390:dbl, "加标回收率"=w388:dbl)
        n218 = Index Array(array=w386, index #1=6 ("索引")) -> (element #1=w392:refnum<vi>, element #2=w389:refnum<vi>)  [unwired: 1 in]
        n219 = property class="DigNum (严格)"(reference=w392, "Value"=w390) -> ()  [unwired: 1 in, 2 out]
        n220 = property class="DigNum (严格)"(reference=w389, "Value"=w388) -> ()  [unwired: 1 in, 2 out]
      }
      event "手动调试": Value Change {
        n221 = event-data() -> ()  [unwired: 1 in, 6 out]
        n222 = call "手动调试界面.vi"() -> ()  [unwired: 16 in]
      }
      event "流程读写": Value Change {
        n223 = event-data() -> ()  [unwired: 1 in, 6 out]
        n224 = call "固定站质控流程参数读取对话框.vi"() -> ()  [unwired: 12 in]
      }
      event "柱塞泵调试": Value Change {
        n225 = event-data() -> ()  [unwired: 1 in, 6 out]
        n226 = call "柱塞泵调试界面.vi"() -> ()  [unwired: 16 in]
      }
      event "打开串口": Value Change {
        n227 = event-data() -> ()  [unwired: 1 in, 6 out]
        n228 = global read "断电保存全局.vi" "MB通信方式选择"() -> (w405:enum16{"串口", "TCP"})
        n229 = global read "断电保存全局.vi" "VISA Resource"() -> (w406:refnum<visa-resource-name>)
        n230 = global read "断电保存全局.vi" "PORT"() -> (w407:string)
        n231 = global read "断电保存全局.vi" "IP"() -> (w408:string)
        n232 = call "串口配置.vi"("PORT"=w407, "IP"=w408, "MB通信方式选择"=w405, "请选择串口:"=w406) -> ("PORT 2"=w412:string, "IP 2"=w413:string, "确认 2"=w415:bool, "VISA资源名称 2"=w414:refnum<visa-resource-name>, "MB通信方式选择 2"=w411:enum16{"串口", "TCP"})  [unwired: 3 in]
        n233 = case shown="真" w415 {
          tunnel: w414 -> [_ w421]
          tunnel: w410 -> [_ w420]
          tunnel: w413 -> [_ w419]
          tunnel: w412 -> [_ w418]
          tunnel: w411 -> [_ w417]
          tunnel: w409 -> [_ w416]
          frame False {
          }
          frame True {
            n234 = flat-sequence {
              tunnel: w421 -> [w425]
              tunnel: w420 -> [w427]
              tunnel: w419 -> [w424]
              tunnel: w418 -> [w423]
              tunnel: w417 -> [w422]
              tunnel: w416 -> [w426]
              frame #0 {
                n235 = global write "断电保存全局.vi" "IP"(w424) -> ()
                n236 = global write "断电保存全局.vi" "PORT"(w423) -> ()
                n237 = global write "断电保存全局.vi" "VISA Resource"(w425) -> ()
                n238 = global write "断电保存全局.vi" "MB通信方式选择"(w422) -> ()
                n239 = Enqueue Element(queue=w427, element=cluster{"命令":string} {"命令"="启用模块"} ("元素"), error in (no error)=w426) -> ()  [unwired: 1 in, 3 out]
              }
              frame #1 {
                n240 = call "配置文件保存.vi"() -> ()  [unwired: 12 in]
              }
            }
          }
        }
      }
      event "释放串口": Value Change {
        n241 = event-data() -> ()  [unwired: 1 in, 6 out]
        n242 = Two Button Dialog(message="确认是否释放串口，释放串口将导致通信失败！" ("消息")) -> (T button?=w431:bool)  [unwired: 2 in]
        n243 = case shown="真" w431 {
          tunnel: w430 -> [_ w434]
          tunnel: w429 -> [_ w433]
          frame False {
          }
          frame True {
            n244 = Bundle By Name(cluster=cluster{"命令":string} {"命令"=""} ("元素"), "命令"="停用模块" ("名称（未命名）")) -> (w435:cluster{"命令":string})
            n245 = Enqueue Element(queue=w434, element=w435, error in (no error)=w433) -> ()  [unwired: 1 in, 3 out]
          }
        }
      }
      event "加标回收": Value Change {
        n246 = event-data() -> ()  [unwired: 1 in, 6 out]
        n247 = Send Notification(notification=FALSE ("通知"), notifier=w446) -> ()  [unwired: 1 in, 2 out]
        n248 = call "质控启动整机或单模块流程对话框.vi"() -> ("确定启动"=w438:bool, "启动模块"=w444:T9, "直接启动"=w441:bool, "常规启动"=w442:bool)  [unwired: 8 in]
        n249 = Not(x=w441) -> (.not. x?=w439:bool)
        n250 = Not(x=w442) -> (.not. x?=w440:bool)
        n251 = Compound Arithmetic op=AND ("复合运算")(w440, w439, w438) -> (w443:bool)
        n252 = case shown="真" w443 {
          tunnel: w444 -> [w450 w468]
          tunnel: w438 -> [w449 _]
          tunnel: w441 -> [w448 _]
          tunnel: w442 -> [w447 _]
          frame False {
            # "整机启动"
            n253 = case shown="真" w449 {
              tunnel: w450 -> [_ w459]
              tunnel: w447 -> [_ w458]
              tunnel: w448 -> [_ w457]
              frame False {
                # "取消启动"
              }
              frame True {
                # "常规或直接启动"
                n254 = Bundle By Name(cluster=T5 {"是否启用仪器"=FALSE, "CODMn"={"启动测量模式"={"测量模式"=enum."水样测量"}, "确定按钮"=FALSE}, "启动模块"={"氨氮"=FALSE, "总磷"=FALSE, "总氮"=FALSE, "CODMn"=FALSE, "CODCr"=FALSE}, "常规启动"=FALSE, "直接启动"=FALSE} ("参数"), "是否启用仪器"=TRUE, "启动模块"=w459, "常规启动"=w458, "直接启动"=w457) -> (w451:T5)
                n255 = vi-ref "流程汇总.vi"() -> (w453:refnum<vi>)
                n256 = property class="VI"(reference=w453) -> ("Name"=w454:string, "Exec.State"=w452:T10)  [unwired: 1 in, 2 out]
                n257 = case shown="\"Idle\"" w452 {
                  tunnel: w454 -> [_ w466 _ _]
                  tunnel: w451 -> [_ w460 _ _]
                  frame "Bad", Default {
                  }
                  frame "Idle" {
                    n258 = Open VI Reference(type specifier VI Refnum (for type only)=refnum<vi> refnum ("类型说明符VI引用句柄（仅用于类型）"), vi path=w466, options=128 ("选项")) -> (vi reference=w467:refnum<vi>, error out=w463:errorcluster)  [unwired: 3 in]
                    n259 = call-by-ref "开始异步调用"(reference=w467, error in=w463, "参数"=w460) -> (reference out=w465:refnum<vi>, error out=w464:errorcluster)  [unwired: 11 in]
                    n260 = Close Reference(reference=w465, error in (no error)=w464) -> ()  [unwired: 1 out]
                  }
                  frame "Run top level" {
                  }
                  frame "Running" {
                  }
                }
              }
            }
          }
          frame True {
            # "单独启动模块加标流程"
            n261 = vi-ref "质控单元.lvlib:单独启动(子VI).vi"() -> (w470:refnum<vi>)
            n262 = property class="VI"(reference=w470) -> ("Name"=w471:string, "Exec.State"=w469:T10)  [unwired: 1 in, 2 out]
            n263 = case shown="\"Idle\"" w469 {
              tunnel: w471 -> [_ w478 _ _]
              tunnel: w468 -> [_ w472 _ _]
              frame "Bad", Default {
              }
              frame "Idle" {
                n264 = Open VI Reference(type specifier VI Refnum (for type only)=refnum<vi> refnum ("类型说明符VI引用句柄（仅用于类型）"), vi path=w478, options=128 ("选项")) -> (vi reference=w479:refnum<vi>, error out=w475:errorcluster)  [unwired: 3 in]
                n265 = call-by-ref "开始异步调用"(reference=w479, error in=w475, "启动模块"=w472) -> (reference out=w477:refnum<vi>, error out=w476:errorcluster)  [unwired: 11 in]
                n266 = Close Reference(reference=w477, error in (no error)=w476) -> ()  [unwired: 1 out]
              }
              frame "Run top level" {
              }
              frame "Running" {
              }
            }
          }
        }
      }
      event "报警清除", "质控流程中": Value Change {
        n267 = event-data() -> ("CtlRef"=w483:refnum<vi>)  [unwired: 1 in, 5 out]
        n268 = property class="Bool"(reference=w483) -> (reference out=w481:refnum<vi>, "Label.Text"=w482:string)  [unwired: 1 in, 1 out]
        n269 = case shown="\"质控流程中\", 默认" w482 {
          tunnel: w481 -> [_ _]
          tunnel: [w484 TRUE ("质控流程中")] -> w480
          frame "质控流程中", Default {
            n270 = local read "质控流程中"() -> (w484:bool)
          }
          frame "报警清除" {
          }
        }
        n271 = case shown="真" w480 {
          frame False {
          }
          frame True {
            w486 = u16 259 ("starting address")
            w492 = FALSE ("氨氮中断报警")
            n272 = global write "质控中断报警全局.vi" "氨氮中断报警"(w492) -> ()
            n273 = global write "质控中断报警全局.vi" "CODMn中断报警"(w492) -> ()
            n274 = global write "质控中断报警全局.vi" "总氮中断报警"(w492) -> ()
            n275 = global write "质控中断报警全局.vi" "总磷中断报警"(w492) -> ()
            n276 = global write "质控中断报警全局.vi" "CODCr中断报警"(w492) -> ()
            n277 = local read "氨氮模块"() -> (w496:bool)
            n278 = case shown="真" w496 {
              tunnel: [errorcluster {"status"=FALSE, "code"=0, "source"=""} ("error out") w521] -> w493
              tunnel: w486 -> [_ w520]
              frame False {
              }
              frame True {
                n279 = call "单个写入.vi"("value"=u16 0, "address"=w520, "Slave ID"=u8 1) -> ("error out"=w521:errorcluster)  [unwired: 8 in]
              }
            }
            n280 = local read "总磷模块选择"() -> (w495:bool)
            n281 = case shown="真" w495 {
              tunnel: w493 -> [w513 w516]
              tunnel: [w513 w515] -> w488
              tunnel: w486 -> [_ w514]
              frame False {
              }
              frame True {
                n282 = call "单个写入.vi"("Error in"=w516, "value"=u16 0, "address"=w514, "Slave ID"=u8 2) -> ("error out"=w515:errorcluster)  [unwired: 7 in]
              }
            }
            n283 = local read "总氮模块选择"() -> (w489:bool)
            n284 = case shown="真" w489 {
              tunnel: w488 -> [w497 w500]
              tunnel: [w497 w499] -> w487
              tunnel: w486 -> [_ w498]
              frame False {
              }
              frame True {
                n285 = call "单个写入.vi"("Error in"=w500, "value"=u16 0, "address"=w498, "Slave ID"=u8 3) -> ("error out"=w499:errorcluster)  [unwired: 7 in]
              }
            }
            n286 = local read "CODMn选择"() -> (w494:bool)
            n287 = case shown="真" w494 {
              tunnel: w487 -> [w507 w510]
              tunnel: [w507 w509] -> w490
              tunnel: w486 -> [_ w508]
              frame False {
              }
              frame True {
                n288 = call "单个写入.vi"("Error in"=w510, "value"=u16 0, "address"=w508, "Slave ID"=u8 4) -> ("error out"=w509:errorcluster)  [unwired: 7 in]
              }
            }
            n289 = local read "CODCr选择"() -> (w491:bool)
            n290 = case shown="真" w491 {
              tunnel: w490 -> [_ w504]
              tunnel: w486 -> [_ w503]
              frame False {
              }
              frame True {
                n291 = call "单个写入.vi"("Error in"=w504, "value"=u16 0, "address"=w503, "Slave ID"=u8 5) -> ()  [unwired: 7 in, 1 out]
              }
            }
          }
        }
      }
      event "平行样测试": Value Change {
        n292 = event-data() -> ()  [unwired: 1 in, 6 out]
        n293 = Cancel Notification(0:w527) -> ()  [unwired: 1 in, 3 out]
        n294 = call "平行样启动流程对话框.vi"() -> ("启动模块"=w526:T11, "常规启动"=w524:bool, "确定启动"=w525:bool)  [unwired: 9 in]
        n295 = case shown="真" w525 {
          tunnel: w526 -> [_ w534]
          tunnel: w524 -> [_ w529]
          frame False {
          }
          frame True {
            n296 = Bundle By Name(cluster=T6 {"参数启用"={"CODMn"=FALSE, "总磷"=FALSE, "总氮"=FALSE, "氨氮"=FALSE, "CODcr"=FALSE}, "采配水是否启动"=FALSE} ("参数"), "参数启用"=w534, "采配水是否启动"=w529) -> (w528:T6)
            n297 = vi-ref "质控单元.lvlib:平行样流程汇总.vi"() -> (w532:refnum<vi>)
            n298 = property class="VI"(reference=w532) -> ("Name"=w533:string, "Exec.State"=w531:T10)  [unwired: 1 in, 2 out]
            n299 = case shown="\"Idle\"" w531 {
              tunnel: w533 -> [_ w541]
              tunnel: w528 -> [_ w535]
              frame "Bad", Default {
              }
              frame "Idle" {
                n300 = Open VI Reference(type specifier VI Refnum (for type only)=refnum<vi> refnum ("类型说明符VI引用句柄（仅用于类型）"), vi path=w541, options=128 ("选项")) -> (vi reference=w542:refnum<vi>, error out=w540:errorcluster)  [unwired: 3 in]
                n301 = call-by-ref "开始异步调用"(reference=w542, error in=w540, "参数"=w535) -> (reference out=w537:refnum<vi>, error out=w536:errorcluster)  [unwired: 11 in]
                n302 = Close Reference(reference=w537, error in (no error)=w536) -> ()  [unwired: 1 out]
              }
            }
          }
        }
      }
      event "停止测量": Value Change {
        w545 = TRUE ("氨氮")
        # "停止采配水、氨氮、总磷总氮、COD、质控"
        n303 = event-data() -> ()  [unwired: 1 in, 6 out]
        n304 = call "质控启动参数选择对话框.vi"("CODCr"=w545, "CODMn"=w545, "总氮"=w545, "总磷"=w545, "氨氮"=w545) -> ("确定启动"=w546:bool, "启动模块"=w547:T9)  [unwired: 4 in, 1 out]
        n305 = case shown="真" w546 {
          tunnel: w547 -> [_ w557]
          tunnel: w544 -> [_ w550]
          tunnel: w543 -> [_ w548]
          frame False {
          }
          frame True {
            n306 = Send Notification(notification=TRUE ("通知"), notifier=w548) -> ()  [unwired: 1 in, 2 out]
            n307 = Unbundle By Name(w557) -> ("氨氮"=w555:bool, "总磷"=w553:bool, "总氮"=w552:bool, "CODMn"=w556:bool, "CODCr"=w554:bool)
            n308 = Enqueue Element At Opposite End(queue=w550, element=T7 {"命令"="单个写入", {"starting address"=300, "holding register value"=2}} ("元素")) -> ()  [unwired: 2 in, 3 out]
            n309 = case shown="真" w553 {
              frame False {
              }
              frame True {
                n310 = call "加标仪器启动命令 (子VI).vi"("启动命令"=enum16{"启动水样流程", "启动加标流程", "排液", "停止"}."停止", "仪器"=enum16{"", "氨氮", "总磷", "总氮", "CODMn", "CODCr"}."总磷") -> ()  [unwired: 9 in, 1 out]
                n311 = Obtain Queue(name (unnamed)="TP" ("名称（未命名）"), element data type=cluster{"命令":string, "data":variant} {"命令"="", "data"=variant}) -> (queue out=w598:refnum<queue>, error out=w588:errorcluster)  [unwired: 3 in, 1 out]
                n312 = Obtain Notifier(name (unnamed)="TP" ("名称（未命名）"), notification data type=FALSE) -> (notifier out=w594:refnum<notifier>, error out=w587:errorcluster)  [unwired: 2 in, 1 out]
                n313 = Send Notification(notification=TRUE ("通知"), notifier=w594, error in (no error)=w587) -> (notifier out=w586:refnum<notifier>, error out=w585:errorcluster)
                n314 = Enqueue Element(queue=w598, element=cluster{"命令":string, "data":variant} {"命令"="启动", "data"=variant(cluster{"站号":u16, "控制命令输出":u16[]} {"站号"=1, "控制命令输出"=[2816]})} ("元素"), error in (no error)=w588) -> (queue out=w583:refnum<queue>, error out=w584:errorcluster)  [unwired: 1 in, 1 out]
                n315 = Release Notifier(notifier=w586, error in (no error)=w585) -> ()  [unwired: 1 in, 3 out]
                n316 = Release Queue(queue=w583, error in (no error)=w584) -> ()  [unwired: 1 in, 3 out]
              }
            }
            n317 = case shown="真" w552 {
              frame False {
              }
              frame True {
                n318 = call "加标仪器启动命令 (子VI).vi"("启动命令"=enum16{"启动水样流程", "启动加标流程", "排液", "停止"}."停止", "仪器"=enum16{"", "氨氮", "总磷", "总氮", "CODMn", "CODCr"}."总氮") -> ()  [unwired: 9 in, 1 out]
                n319 = Obtain Queue(name (unnamed)="TN" ("名称（未命名）"), element data type=cluster{"命令":string, "data":variant} {"命令"="", "data"=variant}) -> (queue out=w573:refnum<queue>, error out=w558:errorcluster)  [unwired: 3 in, 1 out]
                n320 = Obtain Notifier(name (unnamed)="TN" ("名称（未命名）"), notification data type=FALSE) -> (notifier out=w569:refnum<notifier>, error out=w561:errorcluster)  [unwired: 2 in, 1 out]
                n321 = Send Notification(notification=TRUE ("通知"), notifier=w569, error in (no error)=w561) -> (notifier out=w563:refnum<notifier>, error out=w562:errorcluster)
                n322 = Enqueue Element(queue=w573, element=cluster{"命令":string, "data":variant} {"命令"="启动", "data"=variant(cluster{"站号":u16, "控制命令输出":u16[]} {"站号"=1, "控制命令输出"=[2816]})} ("元素"), error in (no error)=w558) -> (queue out=w560:refnum<queue>, error out=w559:errorcluster)  [unwired: 1 in, 1 out]
                n323 = Release Notifier(notifier=w563, error in (no error)=w562) -> ()  [unwired: 1 in, 3 out]
                n324 = Release Queue(queue=w560, error in (no error)=w559) -> ()  [unwired: 1 in, 3 out]
              }
            }
            n325 = case shown="真" w556 {
              frame False {
              }
              frame True {
                n326 = call "CODMn停止命令 (子VI).vi"() -> ()  [unwired: 12 in]
                n327 = Obtain Notifier(name (unnamed)="CODMn" ("名称（未命名）"), notification data type=FALSE) -> (notifier out=w620:refnum<notifier>, error out=w615:errorcluster)  [unwired: 2 in, 1 out]
                n328 = Send Notification(notification=TRUE ("通知"), notifier=w620, error in (no error)=w615) -> (notifier out=w617:refnum<notifier>, error out=w616:errorcluster)
                n329 = call "加标仪器启动命令 (子VI).vi"("启动命令"=enum16{"启动水样流程", "启动加标流程", "排液", "停止"}."停止", "仪器"=enum16{"", "氨氮", "总磷", "总氮", "CODMn", "CODCr"}."CODMn") -> ()  [unwired: 9 in, 1 out]
                n330 = Release Notifier(notifier=w617, error in (no error)=w616) -> ()  [unwired: 1 in, 3 out]
              }
            }
            n331 = case shown="真" w554 {
              frame False {
              }
              frame True {
                n332 = call "CODCr停止命令 (子VI).vi"() -> ()  [unwired: 12 in]
                n333 = Obtain Notifier(name (unnamed)="CODCr" ("名称（未命名）"), notification data type=FALSE) -> (notifier out=w579:refnum<notifier>, error out=w575:errorcluster)  [unwired: 2 in, 1 out]
                n334 = Send Notification(notification=TRUE ("通知"), notifier=w579, error in (no error)=w575) -> (notifier out=w574:refnum<notifier>, error out=w576:errorcluster)
                n335 = call "加标仪器启动命令 (子VI).vi"("启动命令"=enum16{"启动水样流程", "启动加标流程", "排液", "停止"}."停止", "仪器"=enum16{"", "氨氮", "总磷", "总氮", "CODMn", "CODCr"}."CODCr") -> ()  [unwired: 9 in, 1 out]
                n336 = Release Notifier(notifier=w574, error in (no error)=w576) -> ()  [unwired: 1 in, 3 out]
              }
            }
            n337 = case shown="真" w555 {
              frame False {
              }
              frame True {
                n338 = call "加标仪器启动命令 (子VI).vi"("启动命令"=enum16{"启动水样流程", "启动加标流程", "排液", "停止"}."停止", "仪器"=enum16{"", "氨氮", "总磷", "总氮", "CODMn", "CODCr"}."氨氮") -> ()  [unwired: 9 in, 1 out]
                n339 = Obtain Notifier(name (unnamed)="NH3N" ("名称（未命名）"), notification data type=FALSE) -> (notifier out=w610:refnum<notifier>, error out=w604:errorcluster)  [unwired: 2 in, 1 out]
                n340 = Obtain Queue(name (unnamed)="NH3N" ("名称（未命名）"), element data type=cluster{"命令":string, "data":variant} {"命令"="", "data"=variant}) -> (queue out=w614:refnum<queue>, error out=w599:errorcluster)  [unwired: 3 in, 1 out]
                n341 = Send Notification(notification=TRUE ("通知"), notifier=w610, error in (no error)=w604) -> (notifier out=w602:refnum<notifier>, error out=w603:errorcluster)
                n342 = Enqueue Element(queue=w614, element=cluster{"命令":string, "data":variant} {"命令"="启动", "data"=variant(cluster{"站号":u16, "控制命令输出":u16[]} {"站号"=1, "控制命令输出"=[2816]})} ("元素"), error in (no error)=w599) -> (queue out=w601:refnum<queue>, error out=w600:errorcluster)  [unwired: 1 in, 1 out]
                n343 = Release Notifier(notifier=w602, error in (no error)=w603) -> ()  [unwired: 1 in, 3 out]
                n344 = Release Queue(queue=w601, error in (no error)=w600) -> ()  [unwired: 1 in, 3 out]
              }
            }
          }
        }
      }
      event "定时启动": Value Change {
        n345 = event-data() -> ()  [unwired: 1 in, 6 out]
        n346 = flat-sequence {
          frame #0 {
            n347 = global read "断电保存全局.vi" "定时控制"() -> (w624:T12)
            n348 = call "周期设置.vi"("定时控制参数输入"=w624) -> ("定时控制参数输出"=w625:T13)  [unwired: 10 in]
            n349 = global write "断电保存全局.vi" "定时控制"(w625) -> ()
          }
          frame #1 {
            n350 = call "配置文件保存.vi"() -> ()  [unwired: 12 in]
          }
        }
      }
      event "参数设置": Value Change {
        n351 = event-data() -> ()  [unwired: 1 in, 6 out]
        n352 = call "质控参数读取.vi"("section"="氨氮质控参数") -> ("error out"=w659:errorcluster, "参数"=w650:T4)  [unwired: 9 in]
        n353 = Unbundle By Name(w650) -> ("量程"=w647:dbl, "检出限"=w648:dbl, "加标水杯定容体积"=w649:dbl, "加标母液浓度"=w646:dbl)
        n354 = call "质控参数读取.vi"("section"="总磷质控参数", "error in (no error)"=w659) -> ("error out"=w657:errorcluster, "参数"=w645:T4)  [unwired: 8 in]
        n355 = local write "氨氮母液浓度"(w646) -> ()
        n356 = local write "氨氮量程"(w647) -> ()
        n357 = local write "氨氮检出限"(w648) -> ()
        n358 = local write "氨氮加标水杯定容体积"(w649) -> ()
        n359 = Unbundle By Name(w645) -> ("量程"=w644:dbl, "检出限"=w643:dbl, "加标水杯定容体积"=w642:dbl, "加标母液浓度"=w641:dbl)
        n360 = call "质控参数读取.vi"("section"="COD质控参数", "error in (no error)"=w657) -> ("error out"=w655:errorcluster, "参数"=w640:T4)  [unwired: 8 in]
        n361 = local write "总磷检出限"(w643) -> ()
        n362 = local write "总磷量程"(w644) -> ()
        n363 = local write "总磷加标水杯定容体积"(w642) -> ()
        n364 = local write "总磷母液浓度"(w641) -> ()
        n365 = Unbundle By Name(w640) -> ("量程"=w634:dbl, "检出限"=w633:dbl, "加标水杯定容体积"=w632:dbl, "加标母液浓度"=w631:dbl)
        n366 = local write "COD量程"(w634) -> ()
        n367 = local write "COD检出限"(w633) -> ()
        n368 = local write "COD加标水杯定容体积"(w632) -> ()
        n369 = local write "COD母液浓度"(w631) -> ()
        n370 = call "质控参数读取.vi"("section"="总氮质控参数", "error in (no error)"=w655) -> ("error out"=w653:errorcluster, "参数"=w639:T4)  [unwired: 8 in]
        n371 = Unbundle By Name(w639) -> ("量程"=w638:dbl, "检出限"=w637:dbl, "加标水杯定容体积"=w636:dbl, "加标母液浓度"=w635:dbl)
        n372 = local write "总氮量程"(w638) -> ()
        n373 = local write "总氮检出限"(w637) -> ()
        n374 = local write "总氮加标水杯定容体积"(w636) -> ()
        n375 = local write "总氮母液浓度"(w635) -> ()
        n376 = call "质控参数读取.vi"("section"="CODCr质控参数", "error in (no error)"=w653) -> ("error out"=w652:errorcluster, "参数"=w630:T4)  [unwired: 8 in]
        n377 = Unbundle By Name(w630) -> ("量程"=w629:dbl, "检出限"=w628:dbl, "加标水杯定容体积"=w627:dbl, "加标母液浓度"=w626:dbl)
        n378 = local write "CODCr量程"(w629) -> ()
        n379 = local write "CODCr母液浓度"(w626) -> ()
        n380 = local write "CODCr检出限"(w628) -> ()
        n381 = local write "CODCr加标水杯定容体积"(w627) -> ()
        n382 = call <vilib>:"Simple Error Handler.vi"("error in (no error)"=w652) -> ("error out"=w651:errorcluster)  [unwired: 4 in, 4 out]
        n383 = property on="窗格" class="Pane"(error in=w651, "Origin"=T2 {"Horizontal"=0, "Vertical"=640} ("原点")) -> ()  [unwired: 1 in, 2 out]
      }
      event "返回": Value Change {
        n384 = event-data() -> ()  [unwired: 1 in, 6 out]
        n385 = property on="窗格" class="Pane"("Origin"=T2 {"Horizontal"=0, "Vertical"=0} ("原点")) -> ()  [unwired: 2 in, 2 out]
      }
      event "锁定按钮": Value Change {
        n386 = event-data() -> ("NewVal"=w665:bool)  [unwired: 1 in, 5 out]
        n387 = case shown="假" w665 {
          selector: w665 -> [w666 _]
          tunnel: [w666 w667] -> w664
          frame False {
          }
          frame True {
            n388 = call "数字键盘.vi"() -> ("NewNumber"=w670:sgl)  [unwired: 1 in]
            n389 = Equal?(x=w670, y=sgl 23506.0) -> (x = y?=w667:bool)
            n390 = case shown="假" w667 {
              tunnel: ["密码错误！" "解锁成功！"] -> w668
              frame False {
              }
              frame True {
              }
            }
            n391 = One Button Dialog(message=w668) -> ()  [unwired: 1 in, 1 out]
          }
        }
        n392 = local write "解锁？"(w664) -> ()
      }
    }
  }
  n393 = call-by-ref "?"(reference=w71, error in=w73) -> (reference out=w75:refnum<vi>, error out=w74:errorcluster)  [unwired: 12 in]
  n394 = Open VI Reference(type specifier VI Refnum (for type only)=refnum<vi> refnum, vi path=w62, options=128 ("选项")) -> (vi reference=w60:refnum<vi>, error out=w58:errorcluster)  [unwired: 3 in]
  n395 = global write "质控内部交互全局.vi" "配置文件 path"(w14) -> ()
  n396 = call <vilib>:"Open Config Data.vi"("configuration file path"=w14) -> ("error out"=w17:errorcluster, "refnum"=w20:T8)  [unwired: 8 in, 1 out]
  n397 = call-by-ref "?"(reference=w60, error in=w58) -> (reference out=w56:refnum<vi>, error out=w57:errorcluster)  [unwired: 12 in]
  n398 = Close Reference(reference=w75, error in (no error)=w74) -> ()  [unwired: 1 out]
  n399 = call-by-ref "?"(reference=w52, error in=w50, "CODMn"=w44, "总磷"=w45, "CODCr"=w43, "氨氮"=w46, "总氮"=w47) -> (reference out=w48:refnum<vi>, error out=w49:errorcluster)  [unwired: 7 in]
  n400 = vi-ref "质控单元.lvlib:断电保存全局.vi"() -> (w19:refnum<vi>)
  n401 = Close Reference(reference=w56, error in (no error)=w57) -> ()  [unwired: 1 out]
  n402 = Close Reference(reference=w48, error in (no error)=w49) -> ()  [unwired: 1 out]
  n403 = vi-ref "质控单元.lvlib:周期启动 (子VI).vi"() -> (w38:refnum<vi>)
  n404 = call <userlib>:"Read Panel from INI__ogtk.vi"("error in (no error)"=w17, "VI ref"=w19, "refnum"=w20) -> ("error out"=w16:errorcluster, "refnum out"=w18:T8)  [unwired: 7 in]
  n405 = call <vilib>:"Close Config Data.vi"("error in (no error)"=w16, "refnum"=w18) -> ("error out"=w2:errorcluster, "file path"=w4:path)  [unwired: 8 in]
  n406 = Read from Text File(file (use dialog)=w4) -> (text=w13:string, error out=w15:errorcluster)  [unwired: 3 in, 2 out]
  n407 = property class="VI"(reference=w38) -> ("Name"=w37:string)  [unwired: 1 in, 2 out]
  n408 = while {
    tunnel: [w679] -> _
    shift-right: [w677] -> _
    shift-left: w13 -> [w676]
    tunnel: w15 -> [_]
    stop <- FALSE stop-if-true
    n409 = global read "质控内部交互全局.vi" "配置文件 path"() -> (w673:path)
    n410 = Wait (ms)(milliseconds to wait=u32 1000 ("等待时间（毫秒）")) -> ()  [unwired: 1 out]
    n411 = Read from Text File(file (use dialog)=w673) -> (text=w677:string, error out=w674:errorcluster)  [unwired: 3 in, 2 out]
    n412 = Not Equal?(x=w677, y=w676) -> (x != y?=w675:bool)
    n413 = case shown="真" w675 {
      tunnel: [w681 w688] -> w679
      tunnel: w673 -> [_ w682]
      tunnel: w674 -> [w681 _]
      frame False {
      }
      frame True {
        # "文件发生改变进行更新"
        n414 = vi-ref "质控单元.lvlib:断电保存全局.vi"() -> (w683:refnum<vi>)
        n415 = call <vilib>:"Open Config Data.vi"("configuration file path"=w682) -> ("error out"=w687:errorcluster, "refnum"=w686:T8)  [unwired: 8 in, 1 out]
        n416 = call <userlib>:"Read Panel from INI__ogtk.vi"("error in (no error)"=w687, "VI ref"=w683, "refnum"=w686) -> ("error out"=w685:errorcluster, "refnum out"=w684:T8)  [unwired: 7 in]
        n417 = call <vilib>:"Close Config Data.vi"("error in (no error)"=w685, "refnum"=w684) -> ("error out"=w688:errorcluster)  [unwired: 8 in, 1 out]
      }
    }
  }
  n418 = Open VI Reference(type specifier VI Refnum (for type only)=refnum<vi> refnum, vi path=w37, options=128 ("选项")) -> (vi reference=w35:refnum<vi>, error out=w33:errorcluster)  [unwired: 3 in]
  n419 = call-by-ref "?"(reference=w35, error in=w33) -> (reference out=w31:refnum<vi>, error out=w32:errorcluster)  [unwired: 12 in]
  n420 = Close Reference(reference=w31, error in (no error)=w32) -> ()  [unwired: 1 out]
  n421 = while {
    tunnel: w1 -> [_]
    stop <- FALSE stop-if-true
    n422 = local read "模块组合"() -> (w696:enum16{"氨氮总磷", "总磷总氮", "氨氮、总磷、总氮"})
    n423 = Wait (ms)(milliseconds to wait=u32 1000 ("等待时间（毫秒）")) -> ()  [unwired: 1 out]
    n424 = case shown="\"氨氮、总磷、总氮\"" w696 {
      tunnel: ["氨氮总磷模块" "氨氮模块" "氨氮模块"] -> w695
      tunnel: ["总磷模块" "总磷总氮模块" "总磷模块"] -> w694
      tunnel: [u8 1 ("总磷") u8 2 ("总磷") u8 2 ("总磷")] -> w691
      tunnel: [u8 3 ("总磷") u8 2 ("总磷") u8 3 ("总磷")] -> w690
      frame "氨氮总磷", Default {
      }
      frame "总磷总氮" {
      }
      frame "氨氮、总磷、总氮" {
      }
    }
    n425 = global read "断电保存全局.vi" "Slave ID"() -> (w692:T14)
    n426 = property on="模块组合" class="Enum (严格)"("Visible"="解锁？") -> ()  [unwired: 2 in, 2 out]
    n427 = property on="适用类型" class="Enum (严格)"("Visible"="解锁？") -> ()  [unwired: 2 in, 2 out]
    n428 = Bundle By Name(cluster=w692, "总磷"=w691, "总氮"=w690) -> (w693:T14)
    n429 = property on="氨氮模块" class="Bool (严格)"("Caption.Text"=w695) -> ()  [unwired: 2 in, 2 out]
    n430 = property on="总磷模块选择" class="Bool (严格)"("Caption.Text"=w694) -> ()  [unwired: 2 in, 2 out]
    n431 = global write "断电保存全局.vi" "Slave ID"(w693) -> ()
  }
  n432 = while {
    tunnel: w1 -> [_]
    stop <- FALSE stop-if-true
    n433 = global read "质控测完标志全局 1.vi" "总磷总氮平行样测完标志"() -> (→"氨氮总磷平行样测完标志":bool)
    n434 = global read "水样浓度全局.vi" "CODCr加标前水样浓度"() -> (w713:dbl)
    n435 = local read "CODCr加标前水样浓度"() -> (w712:dbl)
    n436 = global read "质控测完标志全局 1.vi" "COD平行样测完标志"() -> (→"COD平行样测完标志":bool)
    n437 = global read "水样浓度全局.vi" "COD加标前水样浓度"() -> (w724:dbl)
    n438 = local read "总氮加标前水样浓度"() -> (w716:dbl)
    n439 = global read "水样浓度全局.vi" "氨氮加标前水样浓度"() -> (w728:dbl)
    n440 = global read "水样浓度全局.vi" "总磷加标前水样浓度"() -> (w726:dbl)
    n441 = local read "COD加标前水样浓度"() -> (w723:dbl)
    n442 = global read "水样浓度全局.vi" "总氮加标前水样浓度"() -> (w715:dbl)
    n443 = local read "氨氮加标前水样浓度"() -> (w727:dbl)
    n444 = local read "总磷加标前水样浓度"() -> (w725:dbl)
    n445 = Wait (ms)(milliseconds to wait=u32 1000 ("等待时间（毫秒）")) -> ()  [unwired: 1 out]
    n446 = Not Equal?(x=w728, y=w727) -> (x != y?=w722:bool)
    n447 = Not Equal?(x=w726, y=w725) -> (x != y?=w720:bool)
    n448 = Not Equal?(x=w724, y=w723) -> (x != y?=w719:bool)
    n449 = Not Equal?(x=w715, y=w716) -> (x != y?=w714:bool)
    n450 = Not Equal?(x=w713, y=w712) -> (x != y?=w711:bool)
    n451 = Compound Arithmetic op=OR ("复合运算")(w722, w720, w719, w714, w711) -> (w721:bool)
    n452 = case shown="真" w721 {
      frame False {
      }
      frame True {
        n453 = global read "水样浓度全局.vi" "CODCr加标前水样浓度"() -> (w731:dbl)
        n454 = global read "水样浓度全局.vi" "COD加标前水样浓度"() -> (w733:dbl)
        n455 = global read "水样浓度全局.vi" "总氮加标前水样浓度"() -> (w732:dbl)
        n456 = global read "水样浓度全局.vi" "总磷加标前水样浓度"() -> (w734:dbl)
        n457 = global read "水样浓度全局.vi" "氨氮加标前水样浓度"() -> (w735:dbl)
        n458 = property on="总氮加标前水样浓度" class="DigNum (严格)"("Val(Sgnl)"=w732) -> ()  [unwired: 2 in, 2 out]
        n459 = property on="CODCr加标前水样浓度" class="DigNum (严格)"("Val(Sgnl)"=w731) -> ()  [unwired: 2 in, 2 out]
        n460 = property on="COD加标前水样浓度" class="DigNum (严格)"("Val(Sgnl)"=w733) -> ()  [unwired: 2 in, 2 out]
        n461 = property on="总磷加标前水样浓度" class="DigNum (严格)"("Val(Sgnl)"=w734) -> ()  [unwired: 2 in, 2 out]
        n462 = property on="氨氮加标前水样浓度" class="DigNum (严格)"("Val(Sgnl)"=w735) -> ()  [unwired: 2 in, 2 out]
      }
    }
  }
  n463 = while {
    tunnel: w1 -> [_]
    stop <- FALSE stop-if-true
    # "状态显示和全局变量赋值"
    n464 = flat-sequence {
      frame #0 {
        # "赋值给全局变量"
        n465 = local read "CODCr加标回收率"() -> (w862:dbl)
        n466 = local read "CODCr加标体积"() -> (w873:dbl)
        n467 = local read "CODCr母液浓度"() -> (w863:dbl)
        n468 = local read "COD加标回收率"() -> (w861:dbl)
        n469 = local read "总磷加标回收率"() -> (w859:dbl)
        n470 = local read "氨氮加标回收率"() -> (w858:dbl)
        n471 = local read "总氮加标回收率"() -> (w860:dbl)
        n472 = local read "总氮加标体积"() -> (w875:dbl)
        n473 = local read "总氮母液浓度"() -> (w865:dbl)
        n474 = local read "COD加标体积"() -> (w874:dbl)
        n475 = local read "COD母液浓度"() -> (w864:dbl)
        n476 = local read "氨氮加标体积"() -> (w877:dbl)
        n477 = local read "氨氮母液浓度"() -> (w867:dbl)
        n478 = local read "总磷母液浓度"() -> (w866:dbl)
        n479 = local read "总磷加标体积"() -> (w876:dbl)
        n480 = local read "CODCr加标水杯定容体积"() -> (w872:dbl)
        n481 = global read "断电保存全局.vi" "定时控制"() -> (w852:T12)
        n482 = local read "总氮加标水杯定容体积"() -> (w870:dbl)
        n483 = local read "CODCr传感器故障报警"() -> (w853:bool)
        n484 = local read "CODMn液位异常报警"() -> (w854:bool)
        n485 = local read "COD加标水杯定容体积"() -> (w871:dbl)
        n486 = local read "氨氮加标水杯定容体积"() -> (w868:dbl)
        n487 = local read "总磷加标水杯定容体积"() -> (w869:dbl)
        n488 = local read "总氮液位异常报警"() -> (w855:bool)
        n489 = local read "总磷液位异常报警"() -> (w856:bool)
        n490 = local read "氨氮液位异常报警"() -> (w857:bool)
        n491 = global read "断电保存全局.vi" "CODCr选择"() -> (w880:bool)
        n492 = global read "断电保存全局.vi" "氨氮模块"() -> (w879:bool)
        n493 = local write "氨氮模块"(w879) -> ()
        n494 = Unbundle By Name(w852) -> ("定时功能启用"=w851:bool)
        n495 = global write "加标回收状态全局变量.vi" "氨氮加标体积"(w877) -> ()
        n496 = global write "加标回收状态全局变量.vi" "总磷加标回收率"(w859) -> ()
        n497 = global read "断电保存全局.vi" "总氮模块选择"() -> (w882:bool)
        n498 = local write "总氮模块选择"(w882) -> ()
        n499 = global write "加标回收状态全局变量.vi" "CODMn加标体积"(w874) -> ()
        n500 = global read "断电保存全局.vi" "氨氮量程选择"() -> (w885:enum32{"H", "L", "AUTO"})
        n501 = local write "氨氮加标回收"(w885) -> ()
        n502 = global write "加标回收状态全局变量.vi" "CODCr加标回收率"(w862) -> ()
        n503 = global write "加标回收状态全局变量.vi" "氨氮母液浓度"(w867) -> ()
        n504 = global write "加标回收状态全局变量.vi" "总磷母液浓度"(w866) -> ()
        n505 = global write "加标回收状态全局变量.vi" "CODCr加标体积"(w873) -> ()
        n506 = global read "断电保存全局.vi" "CODCr量程选择"() -> (w887:enum32{"H", "L", "AUTO"})
        n507 = local write "CODCr加标回收"(w887) -> ()
        n508 = global read "断电保存全局.vi" "CODMn选择"() -> (w881:bool)
        n509 = local write "CODMn选择"(w881) -> ()
        n510 = global write "加标回收状态全局变量.vi" "CODMn母液浓度"(w864) -> ()
        n511 = global write "加标回收状态全局变量.vi" "总磷加标体积"(w876) -> ()
        n512 = global read "断电保存全局.vi" "CODMn量程选择"() -> (w886:enum32{"H", "L", "AUTO"})
        n513 = local write "CODMn加标回收"(w886) -> ()
        n514 = global write "加标回收状态全局变量.vi" "氨氮加标回收率"(w858) -> ()
        n515 = global write "加标回收状态全局变量.vi" "CODMn加标回收率"(w861) -> ()
        n516 = global write "加标回收状态全局变量.vi" "总氮加标回收率"(w860) -> ()
        n517 = global read "断电保存全局.vi" "总磷模块选择"() -> (w878:bool)
        n518 = local write "总磷模块选择"(w878) -> ()
        n519 = global write "加标回收状态全局变量.vi" "总氮加标体积"(w875) -> ()
        n520 = global read "断电保存全局.vi" "总磷量程选择"() -> (w883:enum32{"H", "L", "AUTO"})
        n521 = local write "总磷加标回收"(w883) -> ()
        n522 = global write "加标回收状态全局变量.vi" "CODCr母液浓度"(w863) -> ()
        n523 = global write "加标回收状态全局变量.vi" "总氮母液浓度"(w865) -> ()
        n524 = global read "断电保存全局.vi" "总氮量程选择"() -> (w884:enum32{"H", "L", "AUTO"})
        n525 = local write "总氮加标回收"(w884) -> ()
        n526 = local write "CODCr选择"(w880) -> ()
        n527 = global write "加标回收状态全局变量.vi" "氨氮加标水杯定容体积"(w868) -> ()
        n528 = global write "加标回收状态全局变量.vi" "总磷加标水杯定容体积"(w869) -> ()
        n529 = global write "加标回收状态全局变量.vi" "总氮加标水杯定容体积"(w870) -> ()
        n530 = global write "加标回收状态全局变量.vi" "CODCr加标水杯定容体积"(w872) -> ()
        n531 = global write "加标回收状态全局变量.vi" "CODMn加标水杯定容体积"(w871) -> ()
        n532 = global write "质控中断报警全局.vi" "CODCr传感器故障报警"(w853) -> ()
        n533 = global write "质控中断报警全局.vi" "CODMn传感器故障报警"(w854) -> ()
        n534 = global write "质控中断报警全局.vi" "总氮传感器故障报警"(w855) -> ()
        n535 = global write "质控中断报警全局.vi" "总磷传感器故障报警"(w856) -> ()
        n536 = global write "质控中断报警全局.vi" "氨氮传感器故障报警"(w857) -> ()
        n537 = global read "断电保存全局.vi" "模块组合"() -> (w850:enum16{"氨氮总磷", "总磷总氮", "氨氮、总磷、总氮"})
        n538 = global read "断电保存全局.vi" "适用类型"() -> (w849:enum16{"固定站", "微站"})
        n539 = local write "定时启动"(w851) -> ()
        n540 = local write "模块组合"(w850) -> ()
        n541 = local write "适用类型"(w849) -> ()
      }
    }
    n542 = flat-sequence {
      frame #0 {
        # "界面状态显示"
        n543 = global read "断电保存全局.vi" "MB通信方式选择"() -> (w830:enum16{"串口", "TCP"})
        n544 = global read "质控测完标志全局 1.vi" "CODCr质控流程中"() -> (w837:bool)
        "CODCr质控流程中" <- w837
        n545 = global read "质控中断报警全局.vi" "CODMn中断报警"() -> (→"CODMn流程中断报警":bool)
        n546 = global read "质控测完标志全局 1.vi" "COD质控流程中"() -> (w836:bool)
        "CODMn质控流程中" <- w836
        n547 = global read "质控中断报警全局.vi" "CODCr中断报警"() -> (→"CODCr流程中断报警":bool)
        n548 = global read "质控测完标志全局 1.vi" "总磷质控流程中"() -> (w835:bool)
        "总磷质控流程中" <- w835
        n549 = global read "质控测完标志全局 1.vi" "总氮质控流程中"() -> (w838:bool)
        "总氮质控流程中" <- w838
        n550 = global read "质控测完标志全局 1.vi" "氨氮质控流程中"() -> (w834:bool)
        "氨氮质控流程中" <- w834
        n551 = global read "质控中断报警全局.vi" "氨氮中断报警"() -> (→"氨氮流程中断报警":bool)
        n552 = global read "质控中断报警全局.vi" "总氮中断报警"() -> (→"总氮流程中断报警":bool)
        n553 = global read "质控中断报警全局.vi" "总磷中断报警"() -> (→"总磷流程中断报警":bool)
        n554 = global read "质控测完标志全局 1.vi" "质控流程中"() -> (w832:bool)
        n555 = global read "质控测完标志全局 1.vi" "质控流程中"() -> (w842:bool)
        n556 = case shown="\"串口\", 默认" w830 {
          tunnel: [w847 w848] -> w829
          frame "串口", Default {
            n557 = global read "断电保存全局.vi" "VISA Resource"() -> (w847:refnum<visa-resource-name>)
          }
          frame "TCP" {
            n558 = global read "断电保存全局.vi" "IP"() -> (w848:string)
          }
        }
        "串口/TCP" <- w829
        n559 = Compound Arithmetic op=OR ("复合运算")(w832, w834, w835, w838, w836, w837) -> (→"质控流程中":bool)
        n560 = Select(t=T15."Disabled and Grayed Out" ("禁用"), s=w842, f=T15."Enabled") -> (s? t:f=w831:T15)
        n561 = property on="平行样测试" class="Bool"("DisabledEnum"=w831) -> ()  [unwired: 2 in, 2 out]
        n562 = property on="加标回收" class="Bool"("DisabledEnum"=w831) -> ()  [unwired: 2 in, 2 out]
        n563 = property on="CODCr状态簇" class="Clust (严格)"("Visible"="隐藏按钮") -> ()  [unwired: 2 in, 2 out]
        n564 = property on="氨氮状态簇" class="Clust (严格)"("Visible"="隐藏按钮") -> ()  [unwired: 2 in, 2 out]
        n565 = property on="总磷状态簇" class="Clust (严格)"("Visible"="隐藏按钮") -> ()  [unwired: 2 in, 2 out]
        n566 = property on="CODMn状态簇" class="Clust (严格)"("Visible"="隐藏按钮") -> ()  [unwired: 2 in, 2 out]
        n567 = property on="总氮状态簇" class="Clust (严格)"("Visible"="隐藏按钮") -> ()  [unwired: 2 in, 2 out]
      }
    }
    n568 = flat-sequence {
      frame #0 {
        n569 = global read "质控内部交互全局.vi" "CODCr通讯状态"() -> (→"CODCr通讯":bool)
        n570 = global read "质控内部交互全局.vi" "CODCr测量状态"() -> (w772:u16[])
        n571 = Index Array(array=w772) -> (element #1=w773:u16, element #2=w768:u16, element #3=w764:u16, element #4=w762:u16, element #5=w759:u16, element #6=w758:u16)  [unwired: 6 in]
        "CODCr状态" <- w773
        n572 = Split Number(x=w762) -> (hi(x)=w761:u8, lo(x)=w760:u8)
        n573 = global write "加标回收状态全局变量.vi" "CODCr状态"(w773) -> ()
        n574 = Equal?(x=w768, y=u16 1) -> (x = y?=→"CODCr传感器状态":bool)
        n575 = Equal?(x=w764, y=u16 1) -> (x = y?=→"CODCr传感器故障报警":bool)
        n576 = Equal?(x=w764, y=u16 2) -> (x = y?=→"CODCr柱塞泵故障报警":bool)
        n577 = Bundle By Name(cluster=T1 {"步骤剩余时间"=0, "当前具体步骤"=enum."加标", " 当前流程"=enum."", "当前小步骤数"=0} ("氨氮状态簇"), "当前流程"=w761, "当前小步骤数"=w760, "步骤剩余时间"=w759, "当前具体步骤"=w758) -> (w756:T1)
        "CODCr状态簇" <- w756
        n578 = global write "加标回收状态全局变量.vi" "CODCr状态簇"(w756) -> ()
      }
    }
    n579 = flat-sequence {
      frame #0 {
        n580 = global read "质控内部交互全局.vi" "总氮通讯状态"() -> (→"总氮通讯":bool)
        n581 = global read "质控内部交互全局.vi" "总氮测量状态"() -> (w752:u16[])
        n582 = Index Array(array=w752) -> (element #1=w751:u16, element #2=w754:u16, element #3=w746:u16, element #4=w742:u16, element #5=w740:u16, element #6=w741:u16)  [unwired: 6 in]
        "总氮状态" <- w751
        n583 = Split Number(x=w742) -> (hi(x)=w744:u8, lo(x)=w743:u8)
        n584 = Bundle By Name(cluster=T1 {"步骤剩余时间"=0, "当前具体步骤"=enum."加标", " 当前流程"=enum."", "当前小步骤数"=0} ("氨氮状态簇"), "当前流程"=w744, "当前小步骤数"=w743, "步骤剩余时间"=w740, "当前具体步骤"=w741) -> (w738:T1)
        "总氮状态簇" <- w738
        n585 = global write "加标回收状态全局变量.vi" "总氮状态"(w751) -> ()
        n586 = Equal?(x=w754, y=u16 1) -> (x = y?=→"总氮液位状态":bool)
        n587 = Equal?(x=w746, y=u16 1) -> (x = y?=→"总氮液位异常报警":bool)
        n588 = Equal?(x=w746, y=u16 2) -> (x = y?=→"总氮柱塞泵故障报警":bool)
        n589 = global write "加标回收状态全局变量.vi" "总氮状态簇"(w738) -> ()
      }
    }
    n590 = flat-sequence {
      frame #0 {
        n591 = global read "质控内部交互全局.vi" "CODMn通讯状态"() -> (→"CODMn通讯":bool)
        n592 = global read "质控内部交互全局.vi" "CODMn测量状态"() -> (w788:u16[])
        n593 = Index Array(array=w788) -> (element #1=w791:u16, element #2=w789:u16, element #3=w782:u16, element #4=w778:u16, element #5=w776:u16, element #6=w777:u16)  [unwired: 6 in]
        "CODMn状态" <- w791
        n594 = Split Number(x=w778) -> (hi(x)=w780:u8, lo(x)=w779:u8)
        n595 = global write "加标回收状态全局变量.vi" "COD状态"(w791) -> ()
        n596 = Equal?(x=w789, y=u16 1) -> (x = y?=→"CODMn液位状态":bool)
        n597 = Equal?(x=w782, y=u16 1) -> (x = y?=→"CODMn液位异常报警":bool)
        n598 = Equal?(x=w782, y=u16 2) -> (x = y?=→"CODMn柱塞泵故障报警":bool)
        n599 = Bundle By Name(cluster=T1 {"步骤剩余时间"=0, "当前具体步骤"=enum."加标", " 当前流程"=enum."", "当前小步骤数"=0} ("氨氮状态簇"), "当前流程"=w780, "当前小步骤数"=w779, "步骤剩余时间"=w776, "当前具体步骤"=w777) -> (w774:T1)
        "CODMn状态簇" <- w774
        n600 = global write "加标回收状态全局变量.vi" "CODMn状态簇"(w774) -> ()
      }
    }
    n601 = flat-sequence {
      frame #0 {
        n602 = global read "质控内部交互全局.vi" "总磷通讯状态"() -> (→"总磷通讯":bool)
        n603 = global read "质控内部交互全局.vi" "总磷测量状态"() -> (w806:u16[])
        n604 = Index Array(array=w806) -> (element #1=w807:u16, element #2=w808:u16, element #3=w800:u16, element #4=w796:u16, element #5=w794:u16, element #6=w795:u16)  [unwired: 6 in]
        "总磷状态" <- w807
        n605 = Split Number(x=w796) -> (hi(x)=w798:u8, lo(x)=w797:u8)
        n606 = Bundle By Name(cluster=T1 {"步骤剩余时间"=0, "当前具体步骤"=enum."加标", " 当前流程"=enum."", "当前小步骤数"=0} ("氨氮状态簇"), "当前流程"=w798, "当前小步骤数"=w797, "步骤剩余时间"=w794, "当前具体步骤"=w795) -> (w792:T1)
        "总磷状态簇" <- w792
        n607 = global write "加标回收状态全局变量.vi" "总磷状态"(w807) -> ()
        n608 = Equal?(x=w808, y=u16 1) -> (x = y?=→"总磷液位状态":bool)
        n609 = Equal?(x=w800, y=u16 1) -> (x = y?=→"总磷液位异常报警":bool)
        n610 = Equal?(x=w800, y=u16 2) -> (x = y?=→"总磷柱塞泵故障报警":bool)
        n611 = global write "加标回收状态全局变量.vi" "总磷状态簇"(w792) -> ()
      }
    }
    n612 = flat-sequence {
      frame #0 {
        n613 = global read "质控内部交互全局.vi" "氨氮通讯状态"() -> (→"氨氮通讯":bool)
        n614 = global read "质控内部交互全局.vi" "氨氮测量状态"() -> (w824:u16[])
        n615 = Index Array(array=w824) -> (element #1=w825:u16, element #2=w827:u16, element #3=w818:u16, element #4=w814:u16, element #5=w812:u16, element #6=w813:u16)  [unwired: 6 in]
        "氨氮状态" <- w825
        n616 = Split Number(x=w814) -> (hi(x)=w816:u8, lo(x)=w815:u8)
        n617 = global write "加标回收状态全局变量.vi" "氨氮状态"(w825) -> ()
        n618 = Bundle By Name(cluster=T1 {"步骤剩余时间"=0, "当前具体步骤"=enum."加标", " 当前流程"=enum."", "当前小步骤数"=0} ("氨氮状态簇"), "当前流程"=w816, "当前小步骤数"=w815, "步骤剩余时间"=w812, "当前具体步骤"=w813) -> (w810:T1)
        "氨氮状态簇" <- w810
        n619 = Equal?(x=w827, y=u16 1) -> (x = y?=→"氨氮液位状态":bool)
        n620 = Equal?(x=w818, y=u16 1) -> (x = y?=→"氨氮液位异常报警":bool)
        n621 = Equal?(x=w818, y=u16 2) -> (x = y?=→"氨氮柱塞泵故障报警":bool)
        n622 = global write "加标回收状态全局变量.vi" "氨氮状态簇"(w810) -> ()
      }
    }
    n623 = Wait (ms)(milliseconds to wait=u32 1000 ("等待时间（毫秒）")) -> ()  [unwired: 1 out]
  }
